vi "BStAT_(Doubles).vi"() -> ()   [LabVIEW 2013]
uses:
  <vilib>/Utility/file.llb/Read From Spreadsheet File (DBL).vi
  <vilib>/Utility/file.llb/Write To Spreadsheet File (I64).vi
panel:
  out "framesPerSecond":u32
  out "serve to point":dbl[](array[numeric])
  in  "Word._Application":refnum<k7>
  out "p2y":dbl[](array[numeric])
  out "p1y":dbl[](array[numeric])
  out "point frames":dbl[](array[numeric])
  out "service frames":dbl[](array[numeric])
  out "comp_p1 2":dbl[](array[numeric])
  out "comp_p2 2":dbl[](array[numeric])
  out "comp_p2":dbl[](array[numeric])
  out "comp_p1":dbl[](array[numeric])
  out "game":i32[][](array[numeric])
  out "save2_data":dbl[][](array[numeric])
  out "save1_data":dbl[][](array[numeric])
  out "save2":i32[][](array[numeric])
  out "save1":i32[][](array[numeric])
  out "filedata in":dbl[][](array[numeric]) format="%0.3f"
  out "edited\nevents":dbl[][](array[numeric])
  out "edited to play":dbl[](array[numeric])
  out "P2 position":bool
  out "P1 position":bool
  out "p2code":i32
  out "p1code":i32
  out "frames":dbl[](array[numeric])
  out "Events":bool[](array[boolean])
  out "coded data":dbl[][](array[numeric])
  out "frame data":dbl[][](array[numeric])
  out "Score":dbl[][](array[numeric])
  out "OH":bool[](array[boolean])
  out "BH":bool[](array[boolean])
  out "FH":bool[](array[boolean])
  in  "stop":bool
  in  "Tab Control":enum32{"Coding", "Display"}(tab)=enum."Display"
  in  "Name 4":string
  in  "Player 4":bool
  in  "Name 3":string
  in  "Player 3":bool
  in  "Name 2":string
  in  "Player 2":bool
  in  "Name 1":string
  in  "Player 1":bool
  in  "10 6":bool
  in  "10 5":bool
  in  "10 3":bool
  in  "10 4":bool
  in  "10 2":bool
  in  "10":bool
  in  "9 6":bool
  in  "9 5":bool
  in  "9 3":bool
  in  "9 4":bool
  in  "9 2":bool
  in  "9":bool
  in  "5 6":bool
  in  "5 5":bool
  in  "5 3":bool
  in  "5 4":bool
  in  "5 2":bool
  in  "5":bool
  in  "1 6":bool
  in  "1 5":bool
  in  "1 3":bool
  in  "1 4":bool
  in  "1 2":bool
  in  "1":bool
  in  "2 6":bool
  in  "2 5":bool
  in  "2 3":bool
  in  "2 4":bool
  in  "2 2":bool
  in  "2":bool
  in  "3 6":bool
  in  "3 5":bool
  in  "3 3":bool
  in  "3 4":bool
  in  "3 2":bool
  in  "3":bool
  in  "4 6":bool
  in  "4 5":bool
  in  "4 3":bool
  in  "4 4":bool
  in  "4 2":bool
  in  "4":bool
  in  "6 6":bool
  in  "6 5":bool
  in  "6 3":bool
  in  "6 4":bool
  in  "6 2":bool
  in  "6":bool
  in  "7 6":bool
  in  "7 5":bool
  in  "7 3":bool
  in  "7 4":bool
  in  "7 2":bool
  in  "7":bool
  in  "8 6":bool
  in  "8 5":bool
  in  "8 3":bool
  in  "8 4":bool
  in  "8 2":bool
  in  "8":bool
  in  "5":bool
  in  "TCL 3":bool
  in  "BCL 3":bool
  in  "MCL 3":bool
  in  "BCR 3":bool
  in  "MCR  3":bool
  in  "TCR 3":bool
  in  "TCL 2":bool
  in  "BCL 2":bool
  in  "MCL 2":bool
  in  "BCR 2":bool
  in  "MCR 2":bool
  in  "TCR 2":bool
  in  "Drag control":u32(slide) min=400 max=3000 scale=0.0..6446.0
  in  "UNDO":bool
  out "Last coded":i32
  in  "Progress...":i32(slide) min=400 max=3000 scale=0.0..6277.0
  in  "1":bool
  in  "E2":bool
  in  "E1":bool
  in  "Score2":i32
  in  "W2":bool
  in  "W1":bool
  in  "Score1":i32
  in  "Pause 2":bool
  in  "F_Fr":bool
  in  "S_Fr":bool
  out "Video":T1(plugin-control)
  in  "START":bool
  in  "Video file":path caption="Open AVI file"
  in  "Save data":path caption="Save data to file (select folder ONLY)"
  in  "Start Coding":bool
  out "F_frame":u32
  out "S_frame":u32
  in  "playback speed":dbl(slide) step=0.25 scale=0.25..4.0
  in  "fast forward":bool
  in  "TL 2":bool
  in  "BR 2":bool
  in  "BL 2":bool
  in  "BC 2":bool
  in  "MR  2":bool
  in  "MC 2":bool
  in  "ML 2":bool
  in  "TR 2":bool
  in  "TC 2":bool
  in  "TL 3":bool
  in  "BR 3":bool
  in  "BL 3":bool
  in  "BC 3":bool
  in  "MR  3":bool
  in  "MC 3":bool
  in  "ML 3":bool
  in  "TR 3":bool
  in  "TC 3":bool
  in  "Pause 1":bool
  out "coding":i32[][](array[numeric])
  in  "S2":bool
  in  "S1":bool
  in  "2":bool
  in  "3":bool
  in  "4":bool
  in  "Pause 3":bool
  in  "switch sides":bool
  in  "S3":bool
  in  "S4":bool
  in  "Stop and save":bool
  out "Numeric":dbl format="%<%H:%M:%S>t"
  in  "play back":i32(slide)=1 min=0 max=101 scale=0.0..101.0
  out "DISP":T1(plugin-control)
  in  "Vid file":path caption="Open AVI file"
  in  "Data file":path caption="Read data from"
  in  "Tab Control 2":enum32{"Edit ", "Data Display", "Momentum"}(tab)
  in  "5 2":bool
  in  "1 2":bool
  in  "Serve2":bool
  in  "Serve1":bool
  in  "2 2":bool
  in  "3 2":bool
  in  "4 2":bool
  in  "Serve3":bool
  in  "Serve4":bool
  in  "TCL 4":bool
  in  "BCL 4":bool
  in  "MCL 4":bool
  in  "BCR 4":bool
  in  "MCR  4":bool
  in  "TCR 4":bool
  in  "TL 4":bool
  in  "BR 4":bool
  in  "BL 4":bool
  in  "BC 4":bool
  in  "MR  4":bool
  in  "MC 4":bool
  in  "ML 4":bool
  in  "TR 4":bool
  in  "TC 4":bool
  in  "shots":u8(slide)=2 scale=0.0..5.0
  in  "point 2":bool
  in  "Rally":bool
  in  "Write VI":path caption="Write to AVI file"
  in  "before":u8(slide)=2
  in  "Playback Speed":dbl(slide)=1.0 min=0.25 max=30.0 step=0.25 scale=0.25..2.0
  in  "pause":bool
  in  "stop 2":bool
  in  "Playback\nscore":bool
  in  "P2 score":dbl
  in  "P1 score":dbl
  in  "error":bool
  in  "winner":bool
  in  "point 1":bool
  in  "Team1":bool
  in  "Team2":bool
  in  "FH 2":bool
  in  "BH 2":bool
  in  "ST":bool
  in  "CR 2":bool
  in  "clear":bool
  in  "lob":bool
  in  "drive":bool
  in  "smash":bool
  in  "DR defense":bool
  in  "Half Smash":bool
  in  "drop":bool
  in  "net":bool
  in  "OH 2":bool
  in  "Play":bool
  in  "after":u8(slide)=2 scale=0.0..5.0
  in  "write file":bool
  out "Search events":i32(slide) caption="Scaning(events)..." min=400 max=3000 scale=0.0..86.0
  out "Search score":i32(slide) caption="Searching(score)..." min=400 max=3000 scale=0.0..35.0
  out "writing":i32(slide) caption="Writing..." min=400 max=3000 scale=0.0..101.0
  in  "3 shots":bool
  in  "CL defense":bool
  in  "BL defense":bool
  in  "Player 32":bool
  in  "Player 12":bool
  in  "Player 22":bool
  in  "Player 42":bool
  in  "Compare":bool
  in  "2":string(combo)="1"
  in  "1":string(combo)="1"
  in  "save2":string
  in  "save1":string
  in  "save2":bool
  in  "save1":bool
  in  "Percentage":bool
  in  "display\nselection":string(combo)="1"
  in  "To make white":enum32{""}(tab)
  out "p2 23":string
  out "p2 22":string
  out "p2 21":string
  out "p2 20":string
  out "p2 19":string
  out "p2 18":string
  out "p1 15":string
  out "p1 14":string
  out "p1 13":string
  out "p1 12":string
  out "p1 11":string
  out "p1 10":string
  out "p2 17":string
  out "p2 16":string
  out "p2 11":string
  out "p2 10":string
  out "p2 9":string
  out "p2 14":string
  out "p2 13":string
  out "p2 12":string
  out "p2 15":string
  out "p1 5":string
  out "p1 7":string
  out "p1 6":string
  out "p1 4":string
  out "p1 1":string
  out "p1 3":string
  out "p1 2":string
  out "p1 8":string
  out "p1 9":string
  out "player1 2":string[](array[string])=["0", "0", "0", "0", "0", "0", "0", "0", "0", "0"]
  out "P1graph":cluster{dbl[], "array":dbl[]}(graph)={[0.0, nan, 0.0, nan, 0.0, nan, 0.0, nan, 0.0, nan, 0.0, nan, 0.0, nan, 0.0, nan, 0.0], "array"=[1.0, 2.0, 3.0, 4.0, 5.0, 6.0, 7.0, 8.0, 9.0, 10.0, 11.0, 12.0, 13.0, 14.0, 15.0, 16.0, 17.0]}
  out "Player 1":string[](array[string])=["Fore hand", "Back hand", "Over head", "", "Straight", "Cross", "", "Smash", "Half smash", "DRIVE DEF", "BLOCK DEF", "CLEAR DEF", "Drive/Tap", "Lob", "Drop", "Clear", "Net"]
  out "player2 2":string[](array[string])=["0", "0", "0", "0", "0", "0", "0", "0", "0", "0"]
  out "P2graph":cluster{dbl[], "array":dbl[]}(graph)={[0.0, nan, 0.0, nan, 0.0, nan, 0.0, nan, 0.0, nan, 0.0, nan, 0.0, nan, 0.0, nan, 0.0], "array"=[1.0, 2.0, 3.0, 4.0, 5.0, 6.0, 7.0, 8.0, 9.0, 10.0, 11.0, 12.0, 13.0, 14.0, 15.0, 16.0, 17.0]}
  out "Player 2":string[](array[string])=["Fore hand", "Back hand", "Over head", "", "Straight", "Cross", "", "Smash", "Half smash", "DRIVE DEF", "BLOCK DEF", "CLEAR DEF", "Drive/Tap", "Lob", "Drop", "Clear", "Net"]
  out "W1/E1":string[](array[string])=["0", "0"]
  out "W2/E2":string[](array[string])=["0", "0"]
  out "W/E2":string[](array[string])=["Fore hand", "Back hand", "Over head", "", "Strainght", "Cross", "", "Lob", "Clear", "Drive", "Smash", "Defence", "Chop", "Drop", "Net"]
  out "W/E1":string[](array[string])=["Fore hand", "Back hand", "Over head", "", "Strainght", "Cross", "", "Lob", "Clear", "Drive", "Smash", "Defence", "Chop", "Drop", "Net"]
  out "player2_2":string[](array[string])=["0", "0", "0", "", "0", "0"]
  out "player1_2":string[](array[string])=["0", "0", "0", "", "0", "0"]
  out "Player 2_2":string[](array[string])=["Fore hand", "Back hand", "Over head", "", "Strainght", "Cross", "", "Lob", "Clear", "Drive", "Smash", "Defence", "Chop", "Drop", "Net"]
  out "Player 1_2":string[](array[string])=["Fore hand", "Back hand", "Over head", "", "Strainght", "Cross", "", "Lob", "Clear", "Drive", "Smash", "Defence", "Chop", "Drop", "Net"]
  in  "to make white 2":enum32{""}(tab)
  out "Shortest rally length(sec)":dbl format="%#_3g"
  out "Longest rally length(sec)":dbl format="%#_3g"
  out "momentum graph":cluster{dbl[], dbl[]}[](graph)
  out "Score":dbl[](array[numeric])
  out "Average rally length(sec)":dbl format="%#_3g"
  out "Rally length(sec)":dbl format="%#_3g"
  in  "edit video":bool
  in  "REPORT":bool
  # "Strategic Analysis Tool for Badminton"
  # "Position"
  # "Score"
  # "Smash"
  # "Half Smash"
  # "DRIVE Defence"
  # "BLOCK Defence"
  # "CLEAR Defence"
  # "Drive/Tap"
  # "Lob"
  # "Drop"
  # "Clear"
  # "Net"
  # "Overhead"
  # "Straight"
  # "Cross"
  # "Forehand"
  # "Straight"
  # "Cross"
  # "Backhand"
  # "Straight"
  # "Cross"
  # "Shots to Playback"
  # "TEAM / Player"
  # "Position"
  # "Special Events"
  # "Playback interval (s)"
  # "Score"
  # "to"
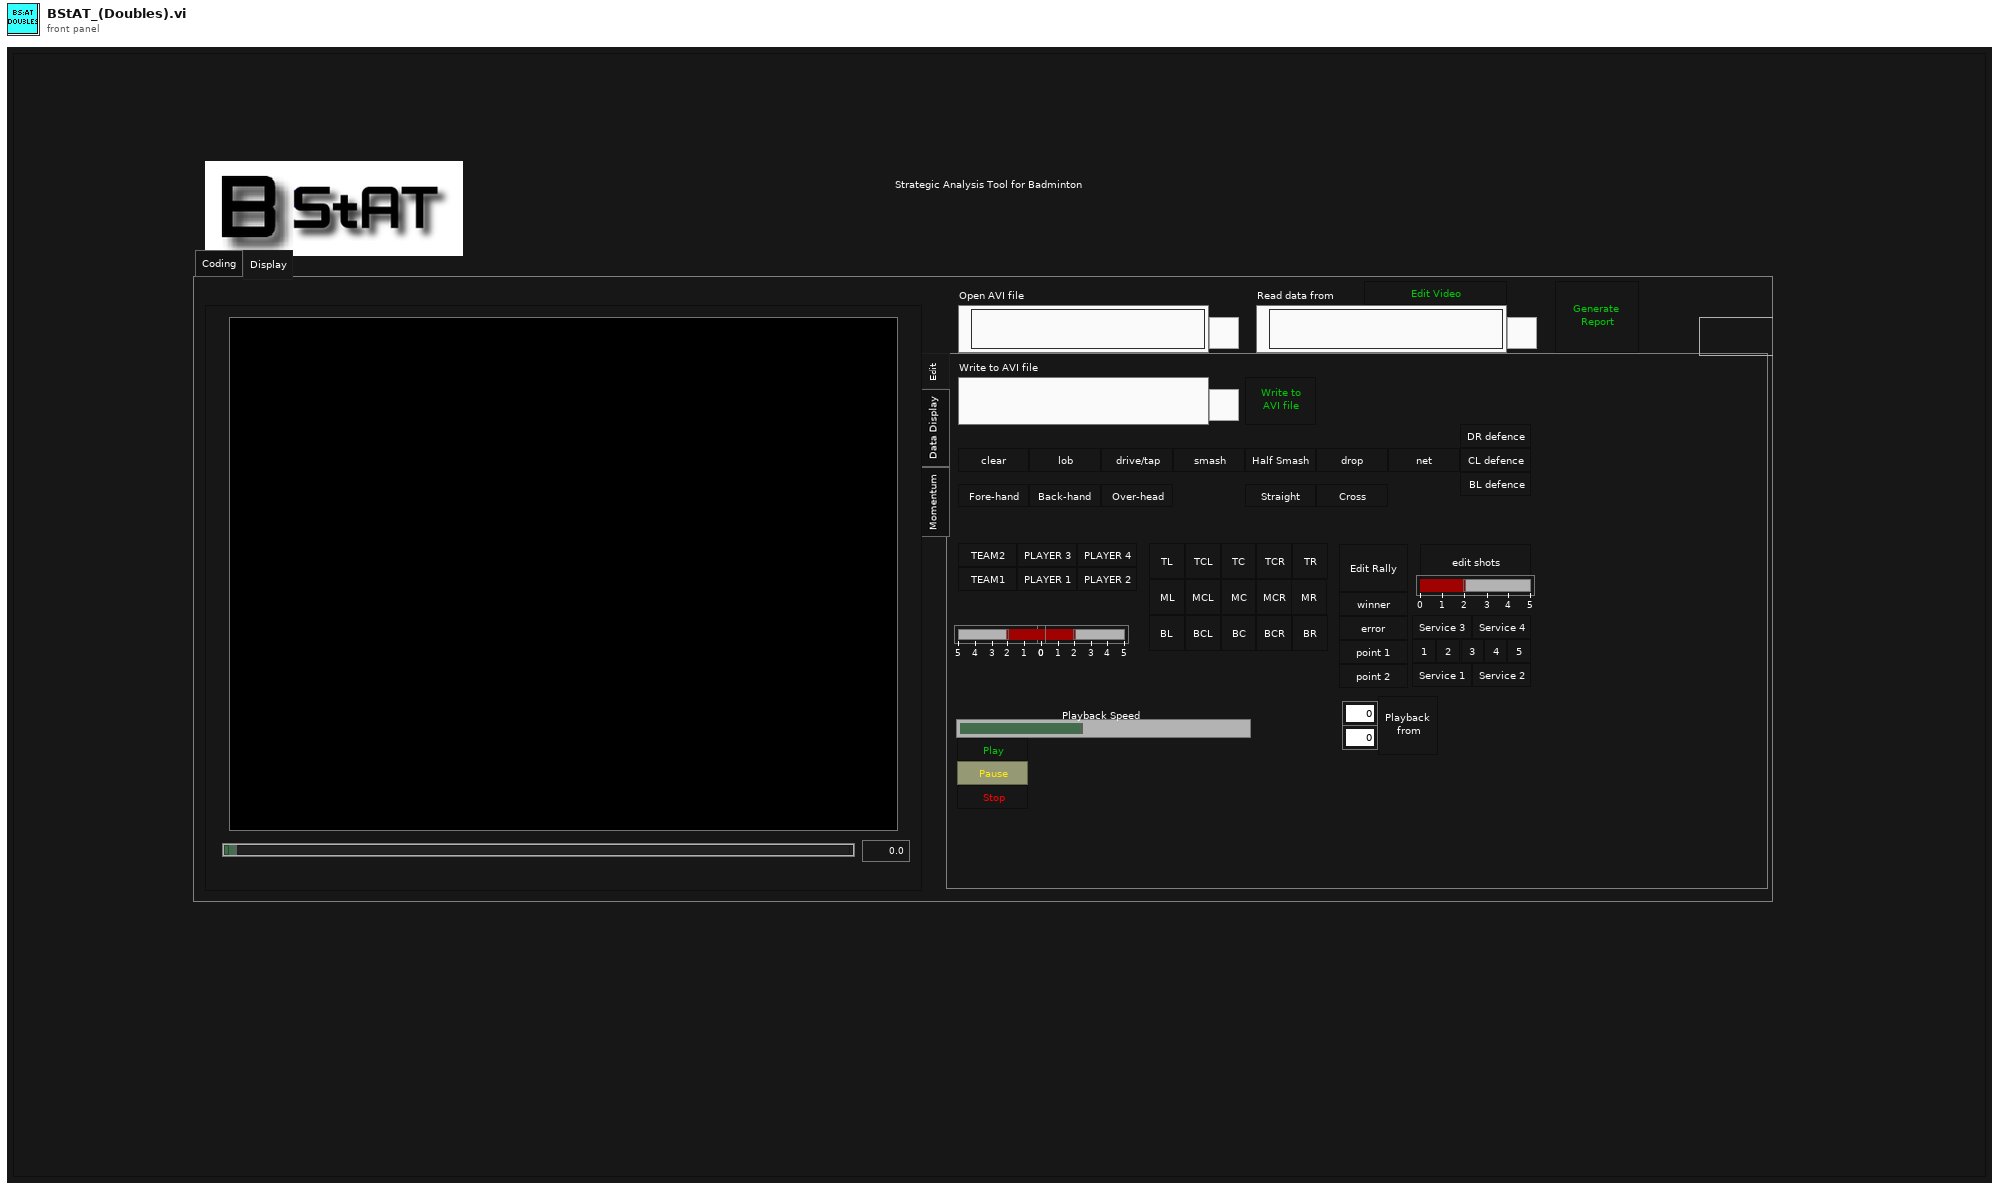
[diagram p1: front panel]
types:
  T1 = typedef "IMAQ Image.ctl" = refnum<image>
  T2 = enum8{"Enabled", "Disabled", "Disabled and Grayed Out"}
  T3 = enum16{"open", "replace", "create", "open or create", "replace or create", "replace or create with confirmation"}
  T4 = typedef "Image Type" = u32
  T5 = typedef "AviRefnum.ctl" = refnum<k1>
  T6 = cluster{"width":u32, "height":u32, "framesPerSecond":u32, "compressionFilter":string, "hasData":bool}
  T7 = typedef "LVPositionTypeDef.ctl" = cluster{"Left":i32, "Top":i32}
  T8 = cluster{"Position":T7, "Position":T7, "Position":T7, "Position":T7, "Position":T7, "Position":T7, "Position":T7, "Position":T7}
  T9 = cluster{"Position":T7, "Position":T7, "Position":T7, "Position":T7, "Position":T7, "Position":T7}
  T10 = cluster{"Position":T7, "Position":T7, "Position":T7, "Position":T7}
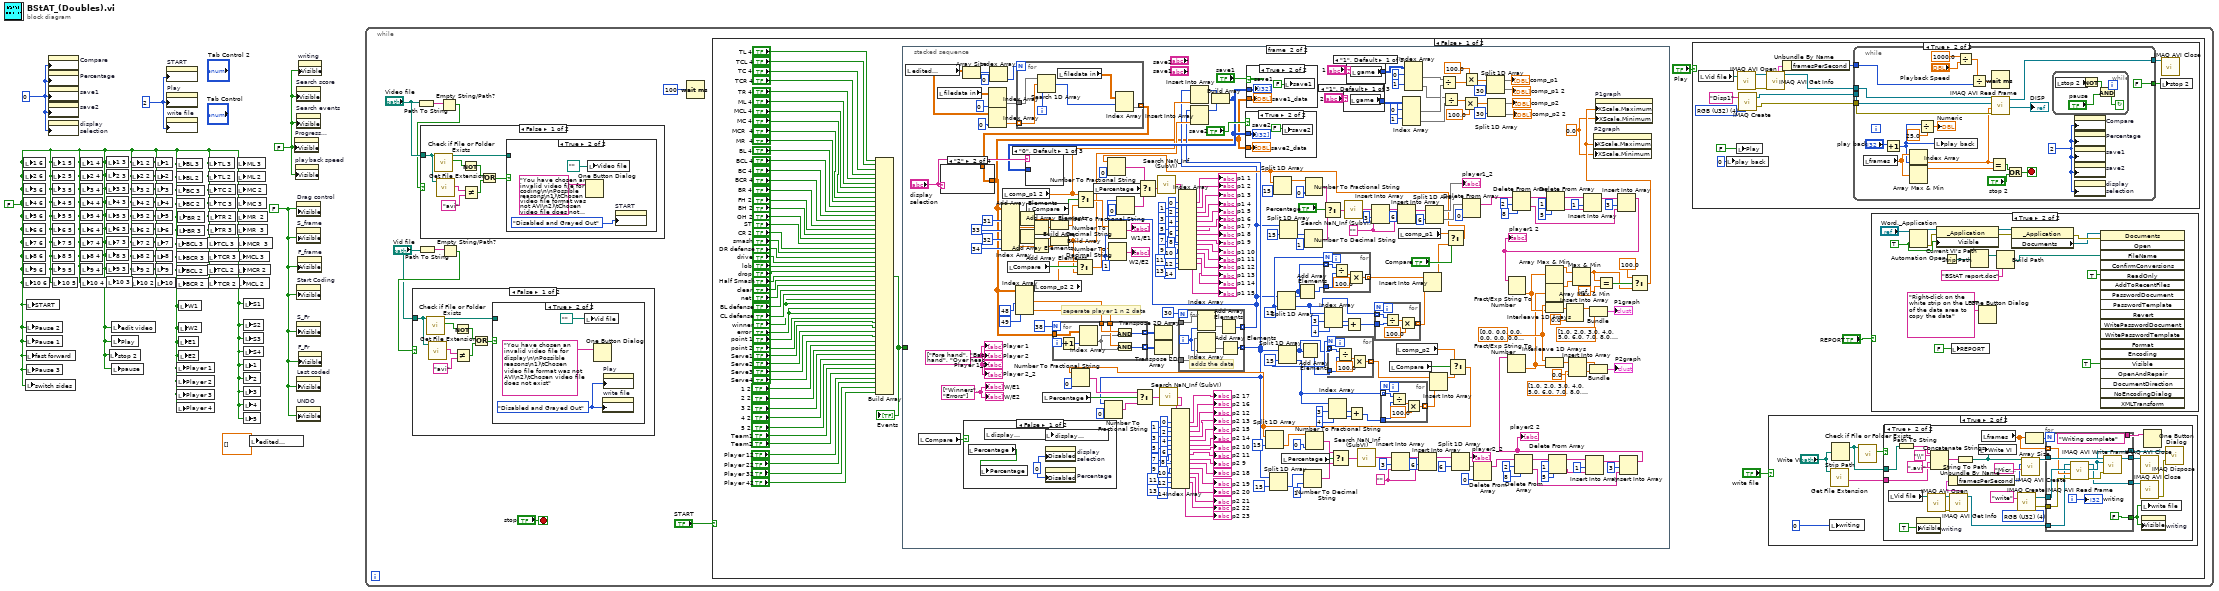
[diagram p0: block diagram]
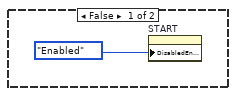
[diagram p2: hidden frame]
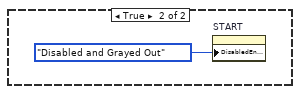
[diagram p3: hidden frame]
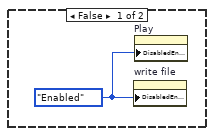
[diagram p4: hidden frame]
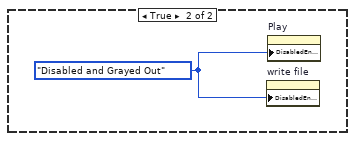
[diagram p5: hidden frame]
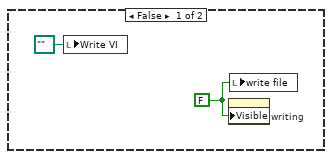
[diagram p7: hidden frame]
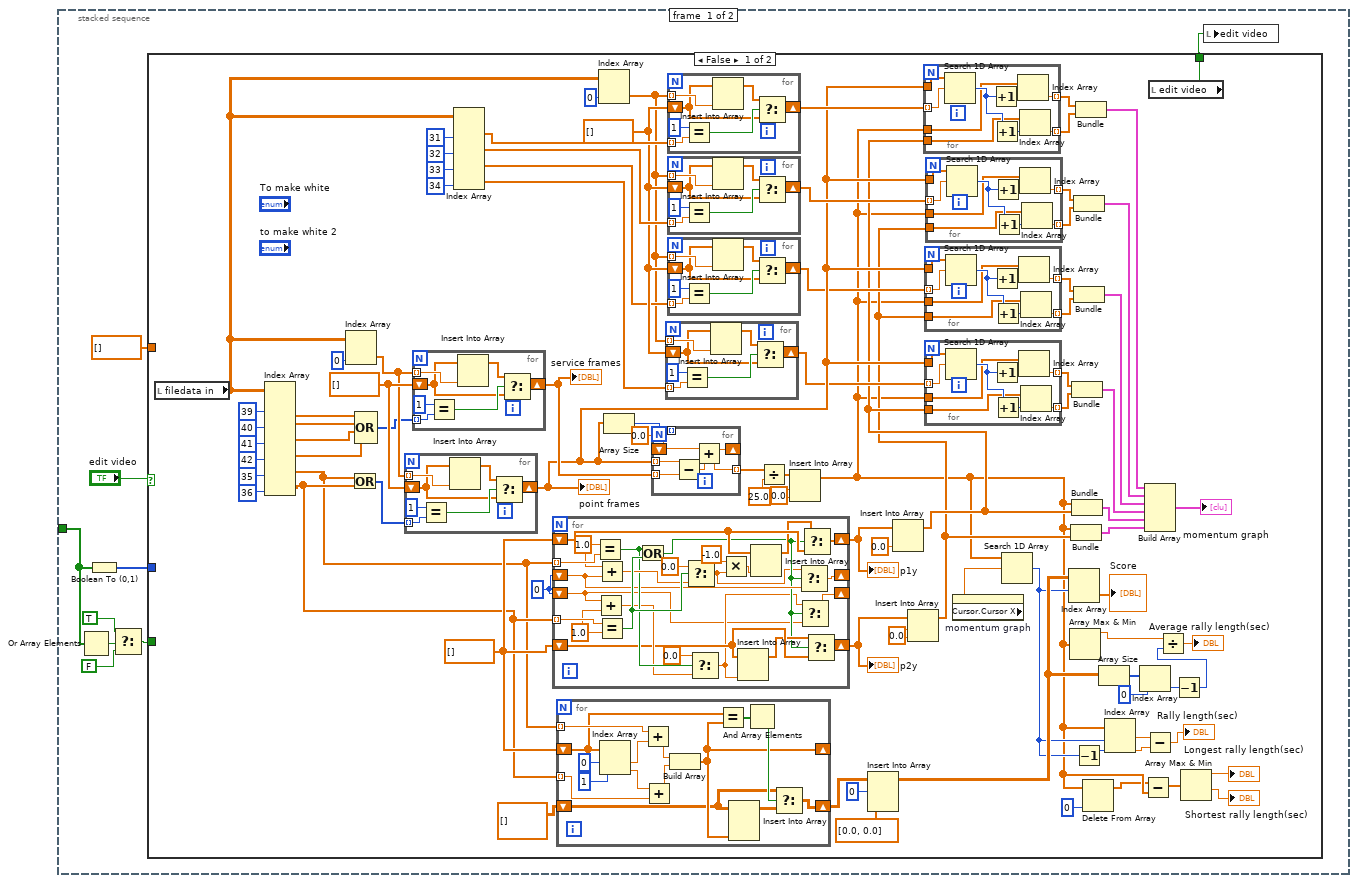
[diagram p9: hidden frame]
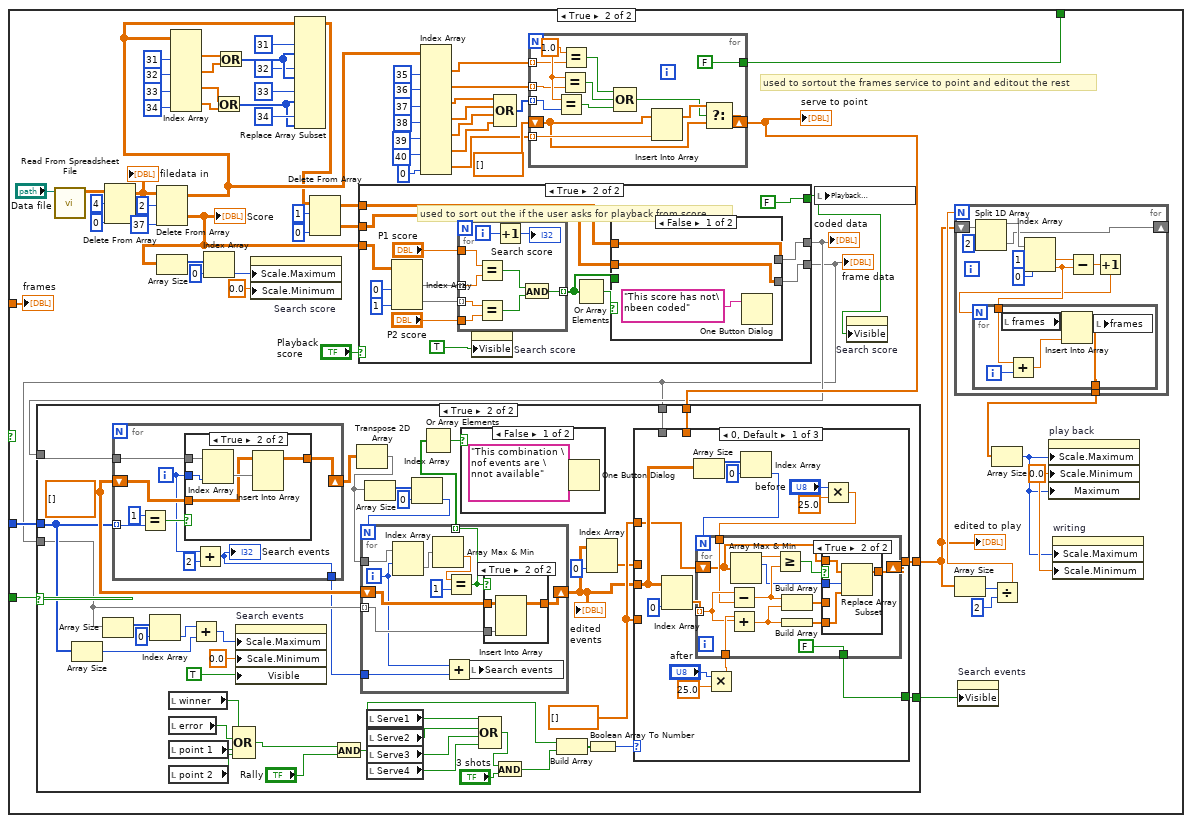
[diagram p10: hidden frame]
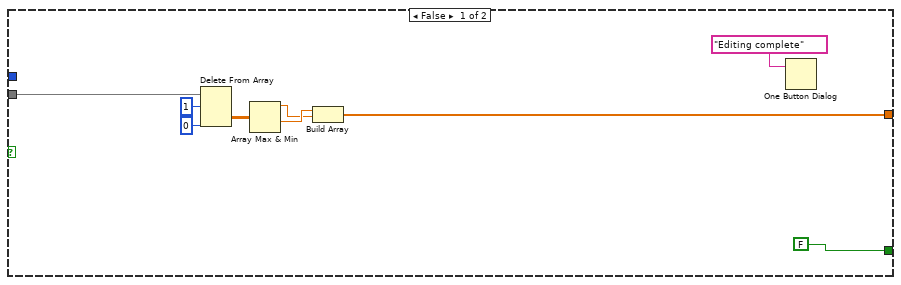
[diagram p11: hidden frame]
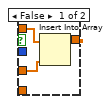
[diagram p12: hidden frame]
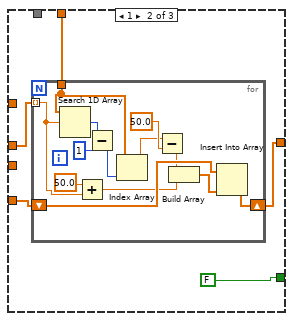
[diagram p13: hidden frame]
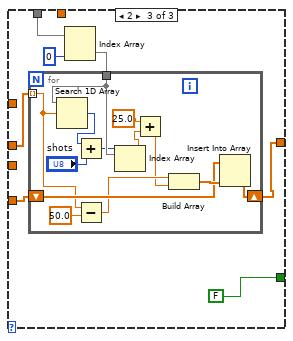
[diagram p14: hidden frame]
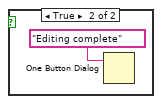
[diagram p15: hidden frame]
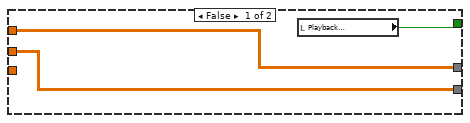
[diagram p18: hidden frame]
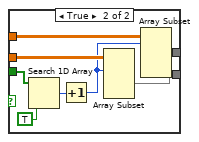
[diagram p19: hidden frame]
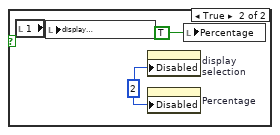
[diagram p20: hidden frame]
diagram:
  w1 = 2 ("play back")
  w2 = 0 ("play back")
  w3 = FALSE ("4 6")
  w4 = FALSE ("Visible")
  w5 = FALSE ("Visible")
  n1 = local write "1 6"(w3) -> ()
  n2 = local write "2 6"(w3) -> ()
  n3 = local write "3 6"(w3) -> ()
  n4 = local write "4 6"(w3) -> ()
  n5 = local write "5 6"(w3) -> ()
  n6 = local write "6 6"(w3) -> ()
  n7 = local write "7 6"(w3) -> ()
  n8 = local write "8 6"(w3) -> ()
  n9 = local write "9 6"(w3) -> ()
  n10 = local write "10 6"(w3) -> ()
  n11 = local write "switch sides"(w3) -> ()
  n12 = local write "START"(w3) -> ()
  n13 = local write "Pause 2"(w3) -> ()
  n14 = local write "Pause 1"(w3) -> ()
  n15 = local write "fast forward"(w3) -> ()
  n16 = local write "Pause 3"(w3) -> ()
  n17 = property on="Compare" class="Bool (strict)"("DisabledEnum"=w2) -> ()  [unwired: 2 in, 2 out]
  n18 = property on="Percentage" class="Bool (strict)"("DisabledEnum"=w2) -> ()  [unwired: 2 in, 2 out]
  n19 = property on="save1" class="Bool (strict)"("DisabledEnum"=w2) -> ()  [unwired: 2 in, 2 out]
  n20 = property on="save2" class="Bool (strict)"("DisabledEnum"=w2) -> ()  [unwired: 2 in, 2 out]
  n21 = property on="display\nselection" class="CmbBox"("DisabledEnum"=w2) -> ()  [unwired: 2 in, 2 out]
  n22 = local write "1 5"(w3) -> ()
  n23 = local write "2 5"(w3) -> ()
  n24 = local write "3 5"(w3) -> ()
  n25 = local write "4 5"(w3) -> ()
  n26 = local write "5 5"(w3) -> ()
  n27 = local write "6 5"(w3) -> ()
  n28 = local write "7 5"(w3) -> ()
  n29 = local write "8 5"(w3) -> ()
  n30 = local write "9 5"(w3) -> ()
  n31 = local write "10 5"(w3) -> ()
  n32 = local write "1 4"(w3) -> ()
  n33 = local write "2 4"(w3) -> ()
  n34 = local write "3 4"(w3) -> ()
  n35 = local write "4 4"(w3) -> ()
  n36 = local write "5 4"(w3) -> ()
  n37 = local write "6 4"(w3) -> ()
  n38 = local write "7 4"(w3) -> ()
  n39 = local write "8 4"(w3) -> ()
  n40 = local write "9 4"(w3) -> ()
  n41 = local write "10 4"(w3) -> ()
  n42 = local write "1 3"(w3) -> ()
  n43 = local write "2 3"(w3) -> ()
  n44 = local write "3 3"(w3) -> ()
  n45 = local write "4 3"(w3) -> ()
  n46 = local write "5 3"(w3) -> ()
  n47 = local write "6 3"(w3) -> ()
  n48 = local write "7 3"(w3) -> ()
  n49 = local write "8 3"(w3) -> ()
  n50 = local write "9 3"(w3) -> ()
  n51 = local write "10 3"(w3) -> ()
  n52 = local write "stop 2"(w3) -> ()
  n53 = local write "edit video"(w3) -> ()
  n54 = local write "Play"(w3) -> ()
  n55 = local write "pause"(w3) -> ()
  n56 = local write "1 2"(w3) -> ()
  n57 = local write "2 2"(w3) -> ()
  n58 = local write "3 2"(w3) -> ()
  n59 = local write "4 2"(w3) -> ()
  n60 = local write "5 2"(w3) -> ()
  n61 = local write "6 2"(w3) -> ()
  n62 = local write "7 2"(w3) -> ()
  n63 = local write "8 2"(w3) -> ()
  n64 = local write "9 2"(w3) -> ()
  n65 = local write "10 2"(w3) -> ()
  n66 = local write "1"(w3) -> ()
  n67 = local write "2"(w3) -> ()
  n68 = local write "3"(w3) -> ()
  n69 = local write "4"(w3) -> ()
  n70 = local write "5"(w3) -> ()
  n71 = local write "6"(w3) -> ()
  n72 = local write "7"(w3) -> ()
  n73 = local write "8"(w3) -> ()
  n74 = local write "9"(w3) -> ()
  n75 = local write "10"(w3) -> ()
  n76 = property on="START" class="Bool (strict)"("DisabledEnum"=w1) -> ()  [unwired: 2 in, 2 out]
  n77 = property on="Play" class="Bool (strict)"("DisabledEnum"=w1) -> ()  [unwired: 2 in, 2 out]
  n78 = property on="write file" class="Bool (strict)"("DisabledEnum"=w1) -> ()  [unwired: 2 in, 2 out]
  n79 = local write "BCL 3"(w3) -> ()
  n80 = local write "BCL 2"(w3) -> ()
  n81 = local write "BL 3"(w3) -> ()
  n82 = local write "BL 2"(w3) -> ()
  n83 = local write "BC 3"(w3) -> ()
  n84 = local write "BC 2"(w3) -> ()
  n85 = local write "BCR 3"(w3) -> ()
  n86 = local write "BCR 2"(w3) -> ()
  n87 = local write "Player 1"(w3) -> ()
  n88 = local write "Player 2"(w3) -> ()
  n89 = local write "Player 3"(w3) -> ()
  n90 = local write "Player 4"(w3) -> ()
  n91 = local write "BR 2"(w3) -> ()
  n92 = local write "BR 3"(w3) -> ()
  n93 = local write "W1"(w3) -> ()
  n94 = local write "W2"(w3) -> ()
  n95 = local write "E1"(w3) -> ()
  n96 = local write "E2"(w3) -> ()
  n97 = local write "TCL 3"(w3) -> ()
  n98 = local write "TCL 2"(w3) -> ()
  n99 = local write "TL 3"(w3) -> ()
  n100 = local write "TL 2"(w3) -> ()
  n101 = local write "TC 2"(w3) -> ()
  n102 = local write "TC 3"(w3) -> ()
  n103 = local write "TCR 3"(w3) -> ()
  n104 = local write "TCR 2"(w3) -> ()
  n105 = local write "TR 2"(w3) -> ()
  n106 = local write "TR 3"(w3) -> ()
  n107 = local write "MCL 3"(w3) -> ()
  n108 = local write "MCL 2"(w3) -> ()
  n109 = local write "ML 3"(w3) -> ()
  n110 = local write "ML 2"(w3) -> ()
  n111 = local write "MC 2"(w3) -> ()
  n112 = local write "MC 3"(w3) -> ()
  n113 = local write "MR  2"(w3) -> ()
  n114 = local write "MR  3"(w3) -> ()
  n115 = local write "MCR  3"(w3) -> ()
  n116 = local write "MCR 2"(w3) -> ()
  n117 = local write "S1"(w3) -> ()
  n118 = local write "S2"(w3) -> ()
  n119 = local write "S3"(w3) -> ()
  n120 = local write "S4"(w3) -> ()
  n121 = local write "1"(w3) -> ()
  n122 = local write "2"(w3) -> ()
  n123 = local write "3"(w3) -> ()
  n124 = local write "4"(w3) -> ()
  n125 = local write "5"(w3) -> ()
  n126 = local write "edited\nevents"(dbl[][] []) -> ()
  n127 = property on="Progress..." class="Slide (strict)"("Visible"=w5) -> ()  [unwired: 2 in, 2 out]
  n128 = property on="playback speed" class="Slide (strict)"("Visible"=w5) -> ()  [unwired: 2 in, 2 out]
  n129 = property on="Search score" class="Slide (strict)"("Visible"=w5) -> ()  [unwired: 2 in, 2 out]
  n130 = property on="Search events" class="Slide (strict)"("Visible"=w5) -> ()  [unwired: 2 in, 2 out]
  n131 = property on="Drag control" class="Slide (strict)"("Visible"=w4) -> ()  [unwired: 2 in, 2 out]
  n132 = property on="S_frame" class="DigNum (strict)"("Visible"=w4) -> ()  [unwired: 2 in, 2 out]
  n133 = property on="Start Coding" class="Bool (strict)"("Visible"=w4) -> ()  [unwired: 2 in, 2 out]
  n134 = property on="S_Fr" class="Bool (strict)"("Visible"=w4) -> ()  [unwired: 2 in, 2 out]
  n135 = property on="Last coded" class="DigNum (strict)"("Visible"=w4) -> ()  [unwired: 2 in, 2 out]
  n136 = property on="UNDO" class="Bool (strict)"("Visible"=w4) -> ()  [unwired: 2 in, 2 out]
  n137 = property on="F_frame" class="DigNum (strict)"("Visible"=w4) -> ()  [unwired: 2 in, 2 out]
  n138 = property on="writing" class="Slide (strict)"("Visible"=w5) -> ()  [unwired: 2 in, 2 out]
  n139 = property on="F_Fr" class="Bool (strict)"("Visible"=w4) -> ()  [unwired: 2 in, 2 out]
  n140 = while {
    stop <- "stop" stop-if-true
    n141 = Path To String(path="Video file") -> (string=w9:string)
    n142 = Path To String(path="Vid file") -> (string=w12:string)
    n143 = Empty String/Path?(string/path=w9) -> (empty?=w7:bool)
    n144 = case shown="False" w7 {
      tunnel: "Video file" -> [w23 _]
      frame False {
        n145 = call <vilib>:"Check if File or Folder Exists.vi"("path"=w23) -> ("file or folder exists?"=w18:bool, "dup path"=w19:path)  [unwired: 8 in, 1 out]
        n146 = call <vilib>:"Get File Extension.vi"("file"=w23) -> ("lowercase file extension"=w22:string)  [unwired: 7 in, 3 out]
        n147 = Not(x=w18) -> (.not. x?=w17:bool)
        n148 = Not Equal?(x=w22, y="avi" ("lowercase file extension")) -> (x != y?=w21:bool)
        n149 = Or(x=w17, y=w21) -> (x .or. y?=w20:bool)
        n150 = case shown="True" w20 {
          tunnel: w19 -> [_ _]
          frame False {
            n151 = property on="START" class="Bool (strict)"("DisabledEnum"=T2."Enabled" ("Disabled")) -> ()  [unwired: 2 in, 2 out]
          }
          frame True {
            n152 = One Button Dialog(message="You have chosen an invalid video file for coding\n\nPossible reasons\n1)\tChosen video file format was not AVI\n2)\tChosen video file does not exist") -> ()  [unwired: 1 in, 1 out]
            n153 = local write "Video file"(path "" ("Video file")) -> ()
            n154 = property on="START" class="Bool (strict)"("DisabledEnum"=T2."Disabled and Grayed Out" ("Disabled")) -> ()  [unwired: 2 in, 2 out]
          }
        }
      }
      frame True {
        n155 = property on="START" class="Bool (strict)"("DisabledEnum"=T2."Disabled and Grayed Out" ("Disabled")) -> ()  [unwired: 2 in, 2 out]
      }
    }
    n156 = Empty String/Path?(string/path=w12) -> (empty?=w11:bool)
    n157 = case shown="False" w11 {
      tunnel: "Vid file" -> [w36 _]
      frame False {
        n158 = call <vilib>:"Check if File or Folder Exists.vi"("path"=w36) -> ("file or folder exists?"=w30:bool, "dup path"=w31:path)  [unwired: 8 in, 1 out]
        n159 = call <vilib>:"Get File Extension.vi"("file"=w36) -> ("lowercase file extension"=w35:string)  [unwired: 7 in, 3 out]
        n160 = Not(x=w30) -> (.not. x?=w29:bool)
        n161 = Not Equal?(x=w35, y="avi" ("lowercase file extension")) -> (x != y?=w33:bool)
        n162 = Or(x=w29, y=w33) -> (x .or. y?=w32:bool)
        n163 = case shown="True" w32 {
          tunnel: w31 -> [_ _]
          frame False {
            w37 = T2."Enabled" ("Disabled")
            n164 = property on="write file" class="Bool (strict)"("DisabledEnum"=w37) -> ()  [unwired: 2 in, 2 out]
            n165 = property on="Play" class="Bool (strict)"("DisabledEnum"=w37) -> ()  [unwired: 2 in, 2 out]
          }
          frame True {
            w39 = T2."Disabled and Grayed Out" ("Disabled")
            n166 = local write "Vid file"(path "" ("Video file")) -> ()
            n167 = One Button Dialog(message="You have chosen an invalid video file for display\n\nPossible reasons\n1)\tChosen video file format was not AVI\n2)\tChosen video file does not exist") -> ()  [unwired: 1 in, 1 out]
            n168 = property on="write file" class="Bool (strict)"("DisabledEnum"=w39) -> ()  [unwired: 2 in, 2 out]
            n169 = property on="Play" class="Bool (strict)"("DisabledEnum"=w39) -> ()  [unwired: 2 in, 2 out]
          }
        }
      }
      frame True {
        w41 = T2."Disabled and Grayed Out" ("Disabled")
        n170 = property on="write file" class="Bool (strict)"("DisabledEnum"=w41) -> ()  [unwired: 2 in, 2 out]
        n171 = property on="Play" class="Bool (strict)"("DisabledEnum"=w41) -> ()  [unwired: 2 in, 2 out]
      }
    }
    n172 = Wait (ms)(milliseconds to wait=u32 100) -> ()  [unwired: 1 out]
    n173 = case shown="False" "START" {
      frame False {
        n174 = Build Array("TL 4", "TCL 4", "TC 4", "TCR 4", "TR 4", "ML 4", "MCL 4", "MC 4", "MCR  4", "MR  4", "BL 4", "BCL 4", "BC 4", "BCR 4", "BR 4", "FH 2", "BH 2", "OH 2", "ST", "CR 2", "smash", "DR defense", "drive", "lob", "drop", "Half Smash", "clear", "net", "BL defense", "CL defense", "winner", "winner", "error", "error", "point 1", "point 2", "Serve1", "Serve2", "Serve3", "Serve4", "1 2", "2 2", "3 2", "4 2", "5 2", "Team1", "Team2", "Player 12", "Player 22", "Player 32", "Player 42") -> (w86:bool[])
        "Events" <- w86
        n175 = stacked-sequence {
          tunnel: w86 -> [w163 _]
          frame #0 {
            n176 = Or Array Elements(Boolean array=w163) -> (logical OR=w166:bool)
            n177 = Boolean To (0,1)(Boolean=w163) -> (0, 1=w162:i16[])
            n178 = Select(t=TRUE, s=w166, f=FALSE) -> (s? t:f=w161:bool)
            n179 = case shown="False" "edit video" {
              tunnel: [w255 w391] -> w159
              tunnel: w162 -> [_ w389]
              tunnel: w161 -> [_ w427]
              tunnel: dbl[] [] ("edited\nto play 3") -> [_ w425]
              frame False {
                w211 = dbl[] []
                w245 = 0.0 ("new element/subarray")
                w244 = 0.0 ("new element/subarray")
                w243 = 0.0 ("new element/subarray")
                w195 = dbl[] []
                w196 = 0 ("disabled index (col)")
                w236 = dbl[] []
                n180 = local read "filedata in"() -> (w212:dbl[][])
                n181 = Index Array(array=w212, index (col) #1=39 ("length"), index (col) #2=40 ("disabled index (col)"), index (col) #3=41 ("index (col)"), index (col) #4=42 ("index (col)"), index (col) #5=35 ("index (col)"), index (col) #6=36 ("index (col)")) -> (element #1=w228:dbl[], element #2=w229:dbl[], element #3=w170:dbl[], element #4=w169:dbl[], element #5=w171:dbl[], element #6=w172:dbl[])  [unwired: 6 in]
                n182 = Index Array(array=w212, index (col)=0 ("disabled index (col)")) -> (element=w235:dbl[])  [unwired: 1 in]
                n183 = Or(x=w171, y=w172) -> (x .or. y?=w234:i32[])
                n184 = Compound Arithmetic op=OR(w228, w229, w170, w169) -> (w231:i32[])
                n185 = for {
                  tunnel: w234 -> [w372] mode=indexing
                  tunnel: w235 -> [w368] mode=indexing
                  shift-right: [w367] -> w207
                  shift-left: w236 -> [w366]
                  n186 = Equal?(x=1, y=w372) -> (x = y?=w370:bool)
                  n187 = Insert Into Array(array=w366, new element=w368) -> (w369:dbl[])  [unwired: 1 in]
                  n188 = Select(t=w369, s=w370, f=w366) -> (s? t:f=w367:dbl[])
                }
                "point frames" <- w207
                n189 = for {
                  tunnel: w231 -> [w379] mode=indexing
                  tunnel: w235 -> [w375] mode=indexing
                  shift-right: [w374] -> w238
                  shift-left: w236 -> [w373]
                  n190 = Equal?(x=1, y=w379) -> (x = y?=w377:bool)
                  n191 = Insert Into Array(array=w373, new element=w375) -> (w376:dbl[])  [unwired: 1 in]
                  n192 = Select(t=w376, s=w377, f=w373) -> (s? t:f=w374:dbl[])
                }
                "service frames" <- w238
                n193 = Index Array(array=w212, index (col) #1=31 ("disabled index (col)"), index (col) #2=32 ("index (col)"), index (col) #3=33 ("index (col)"), index (col) #4=34 ("index (col)")) -> (element #1=w221:dbl[], element #2=w222:dbl[], element #3=w210:dbl[], element #4=w209:dbl[])  [unwired: 4 in]
                n194 = for {
                  shift-right: [w264] -> _
                  shift-left: w196 -> [w263]
                  shift-right: [w260] -> _
                  shift-left: w196 -> [w259]
                  shift-right: [w269] -> w193
                  shift-left: w195 -> [w268]
                  shift-right: [w275] -> w194
                  shift-left: w195 -> [w266]
                  tunnel: w172 -> [w272] mode=indexing
                  tunnel: w171 -> [w280] mode=indexing
                  w271 = 1.0 ("x")
                  w277 = 1.0 ("x")
                  n195 = Equal?(x=w277, y=w280) -> (x = y?=w273:bool)
                  n196 = Add(x=w259, y=w271) -> (x+y=w270:dbl)
                  n197 = Add(x=w277, y=w263) -> (x+y=w276:dbl)
                  n198 = Equal?(x=w272, y=w271) -> (x = y?=w279:bool)
                  n199 = Or(x=w273, y=w279) -> (x .or. y?=w262:bool)
                  n200 = Select(t=0.0, s=w279, f=w276) -> (s? t:f=w256:dbl)
                  n201 = Select(t=0.0, s=w273, f=w270) -> (s? t:f=w261:dbl)
                  n202 = Multiply(x=-1.0 ("y"), y=w256) -> (x*y=w258:dbl)
                  n203 = Insert Into Array(array=w266, new element=w261) -> (w265:dbl[])  [unwired: 1 in]
                  n204 = Insert Into Array(array=w268, new element=w258) -> (w267:dbl[])  [unwired: 1 in]
                  n205 = Select(t=w256, s=w262, f=w263) -> (s? t:f=w264:dbl)
                  n206 = Select(t=w261, s=w262, f=w259) -> (s? t:f=w260:dbl)
                  n207 = Select(t=w267, s=w262, f=w268) -> (s? t:f=w269:dbl[])
                  n208 = Select(t=w265, s=w262, f=w266) -> (s? t:f=w275:dbl[])
                }
                "p1y" <- w193
                "p2y" <- w194
                n209 = for {
                  tunnel: w171 -> [w356] mode=indexing
                  tunnel: w172 -> [w352] mode=indexing
                  shift-right: [w348] -> _
                  shift-left: w195 -> [w351]
                  shift-right: [w346] -> w250
                  shift-left: dbl[][] [] -> [w345]
                  n210 = Index Array(array=w351, index #1=0 ("index"), index #2=1 ("index")) -> (element #1=w357:dbl, element #2=w355:dbl)
                  n211 = Add(x=w356, y=w357) -> (x+y=w354:dbl)
                  n212 = Add(x=w355, y=w352) -> (x+y=w353:dbl)
                  n213 = Build Array(w354, w353) -> (w348:dbl[])
                  n214 = Equal?(x=w351, y=w348) -> (x = y?=w350:bool[])
                  n215 = Insert Into Array(array=w345, new element=w348) -> (w347:dbl[][])  [unwired: 2 in]
                  n216 = And Array Elements(Boolean array=w350) -> (logical AND=w349:bool)
                  n217 = Select(t=w345, s=w349, f=w347) -> (s? t:f=w346:dbl[][])
                }
                n218 = Index Array(array=w212, index (col)=0 ("disabled index (col)")) -> (element=w208:dbl[])  [unwired: 1 in]
                n219 = Array Size(array=w207) -> (size(s)=w237:i32)
                n220 = for {
                  N: w237 -> [w360]
                  tunnel: w207 -> [w365] mode=indexing
                  tunnel: w238 -> [w364] mode=indexing
                  tunnel: [w361] -> w247 mode=indexing
                  shift-right: [w361] -> _
                  shift-left: 0.0 -> [w362]
                  tunnel: [w360] -> _ mode=indexing
                  n221 = Subtract(x=w365, y=w364) -> (x-y=w363:dbl)
                  n222 = Add(x=w362, y=w363) -> (x+y=w361:dbl)
                }
                n223 = for {
                  tunnel: w209 -> [w305] mode=indexing
                  tunnel: w208 -> [w301] mode=indexing
                  shift-right: [w300] -> w205
                  shift-left: w211 -> [w299]
                  n224 = Equal?(x=1, y=w305) -> (x = y?=w303:bool)
                  n225 = Insert Into Array(array=w299, new element=w301) -> (w302:dbl[])  [unwired: 1 in]
                  n226 = Select(t=w302, s=w303, f=w299) -> (s? t:f=w300:dbl[])
                }
                n227 = for {
                  tunnel: w221 -> [w344] mode=indexing
                  tunnel: w208 -> [w340] mode=indexing
                  shift-right: [w339] -> w218
                  shift-left: w211 -> [w338]
                  n228 = Equal?(x=1, y=w344) -> (x = y?=w342:bool)
                  n229 = Insert Into Array(array=w338, new element=w340) -> (w341:dbl[])  [unwired: 1 in]
                  n230 = Select(t=w341, s=w342, f=w338) -> (s? t:f=w339:dbl[])
                }
                n231 = for {
                  tunnel: w222 -> [w337] mode=indexing
                  tunnel: w208 -> [w333] mode=indexing
                  shift-right: [w332] -> w223
                  shift-left: w211 -> [w331]
                  n232 = Equal?(x=1, y=w337) -> (x = y?=w335:bool)
                  n233 = Insert Into Array(array=w331, new element=w333) -> (w334:dbl[])  [unwired: 1 in]
                  n234 = Select(t=w334, s=w335, f=w331) -> (s? t:f=w332:dbl[])
                }
                n235 = for {
                  tunnel: w210 -> [w312] mode=indexing
                  tunnel: w208 -> [w308] mode=indexing
                  shift-right: [w307] -> w206
                  shift-left: w211 -> [w306]
                  n236 = Equal?(x=1, y=w312) -> (x = y?=w310:bool)
                  n237 = Insert Into Array(array=w306, new element=w308) -> (w309:dbl[])  [unwired: 1 in]
                  n238 = Select(t=w309, s=w310, f=w306) -> (s? t:f=w307:dbl[])
                }
                n239 = Divide(x=w247, y=25.0 ("new element/subarray")) -> (x/y=w246:dbl[])
                n240 = Insert Into Array(array=w246, index=w243, new element=w243) -> (w177:dbl[])
                n241 = Insert Into Array(array=w250, index (row)=0, new element=dbl[] [0.0, 0.0] ("new element/subarray")) -> (w190:dbl[][])  [unwired: 1 in]
                n242 = Insert Into Array(array=w193, index=w245, new element=w245) -> (w192:dbl[])
                n243 = Insert Into Array(array=w194, index=w244, new element=w244) -> (w191:dbl[])
                n244 = for {
                  tunnel: w218 -> [w330] mode=indexing
                  tunnel: w207 -> [w329]
                  tunnel: [w327] -> w219 mode=indexing
                  tunnel: [w324] -> w220 mode=indexing
                  tunnel: w177 -> [w323]
                  tunnel: w192 -> [w322]
                  n245 = Search 1D Array(1D array=w329, element=w330) -> (index of element=w325:i32)  [unwired: 1 in]
                  n246 = Increment(x=w325) -> (x+1=w328:i32)
                  n247 = Increment(x=w325) -> (x+1=w326:i32)
                  n248 = Index Array(array=w323, index=w328) -> (element=w327:dbl)
                  n249 = Index Array(array=w322, index=w326) -> (element=w324:dbl)
                }
                n250 = for {
                  tunnel: w206 -> [w298] mode=indexing
                  tunnel: w207 -> [w297]
                  tunnel: [w295] -> w204 mode=indexing
                  tunnel: [w292] -> w203 mode=indexing
                  tunnel: w177 -> [w291]
                  tunnel: w191 -> [w290]
                  n251 = Search 1D Array(1D array=w297, element=w298) -> (index of element=w293:i32)  [unwired: 1 in]
                  n252 = Increment(x=w293) -> (x+1=w296:i32)
                  n253 = Increment(x=w293) -> (x+1=w294:i32)
                  n254 = Index Array(array=w291, index=w296) -> (element=w295:dbl)
                  n255 = Index Array(array=w290, index=w294) -> (element=w292:dbl)
                }
                n256 = for {
                  tunnel: w205 -> [w289] mode=indexing
                  tunnel: w207 -> [w288]
                  tunnel: [w286] -> w202 mode=indexing
                  tunnel: [w283] -> w201 mode=indexing
                  tunnel: w177 -> [w282]
                  tunnel: w192 -> [w281]
                  n257 = Search 1D Array(1D array=w288, element=w289) -> (index of element=w284:i32)  [unwired: 1 in]
                  n258 = Increment(x=w284) -> (x+1=w287:i32)
                  n259 = Increment(x=w284) -> (x+1=w285:i32)
                  n260 = Index Array(array=w282, index=w287) -> (element=w286:dbl)
                  n261 = Index Array(array=w281, index=w285) -> (element=w283:dbl)
                }
                n262 = for {
                  tunnel: w223 -> [w321] mode=indexing
                  tunnel: w207 -> [w320]
                  tunnel: [w318] -> w224 mode=indexing
                  tunnel: [w315] -> w225 mode=indexing
                  tunnel: w177 -> [w314]
                  tunnel: w191 -> [w313]
                  n263 = Search 1D Array(1D array=w320, element=w321) -> (index of element=w316:i32)  [unwired: 1 in]
                  n264 = Increment(x=w316) -> (x+1=w319:i32)
                  n265 = Increment(x=w316) -> (x+1=w317:i32)
                  n266 = Index Array(array=w314, index=w319) -> (element=w318:dbl)
                  n267 = Index Array(array=w313, index=w317) -> (element=w315:dbl)
                }
                n268 = property on="momentum graph" class="XYGraph (strict)"() -> ("Cursor.Cursor X"=w253:dbl)  [unwired: 2 in, 2 out]
                n269 = Search 1D Array(1D array=w177, element=w253) -> (index of element=w182:i32)  [unwired: 1 in]
                n270 = Index Array(array=w190, index (row)=w182) -> (element=→"Score":dbl[])  [unwired: 1 in]
                n271 = Array Max & Min(array=w177) -> (max value=w186:dbl)  [unwired: 3 out]
                n272 = Bundle(w177, w191) -> (w239:cluster{dbl[], dbl[]})  [unwired: 1 in]
                n273 = Bundle(w202, w201) -> (w197:cluster{dbl[], dbl[]})  [unwired: 1 in]
                n274 = Bundle(w177, w192) -> (w240:cluster{dbl[], dbl[]})  [unwired: 1 in]
                n275 = Bundle(w224, w225) -> (w199:cluster{dbl[], dbl[]})  [unwired: 1 in]
                n276 = Bundle(w204, w203) -> (w198:cluster{dbl[], dbl[]})  [unwired: 1 in]
                n277 = Decrement(x=w182) -> (x-1=w183:i32)
                n278 = Bundle(w219, w220) -> (w200:cluster{dbl[], dbl[]})  [unwired: 1 in]
                n279 = Delete From Array(array=w177, index=0) -> (array with subset deleted=w176:dbl[])  [unwired: 1 in, 1 out]
                n280 = Array Size(array=w190) -> (size(s)=w189:i32[])
                n281 = Index Array(array=w177, index #1=w182, index #2=w183) -> (element #1=w180:dbl, element #2=w181:dbl)
                n282 = Index Array(array=w189, index=0) -> (element=w187:i32)
                n283 = Subtract(x=w176, y=w177) -> (x-y=w175:dbl[])
                n284 = Build Array(w200, w199, w198, w197, w240, w239) -> (→"momentum graph":cluster{dbl[], dbl[]}[])
                n285 = Subtract(x=w180, y=w181) -> (x-y=→"Rally length(sec)":dbl)
                n286 = local read "edit video"() -> (w255:bool)
                n287 = Decrement(x=w187) -> (x-1=w185:i32)
                n288 = Divide(x=w186, y=w185) -> (x/y=→"Average rally length(sec)":dbl)
                n289 = Array Max & Min(array=w175) -> (max value=→"Longest rally length(sec)":dbl, min value=→"Shortest rally length(sec)":dbl)  [unwired: 2 out]
              }
              frame True {
                w423 = 0.0 ("Scale.Range:Minimum")
                # "used to sortout the frames service to point and editout the rest"
                n290 = call-poly <vilib>:"Read From Spreadsheet File.vi"("file path (dialog if empty)"="Data file") -> ("all rows"=w441:dbl[][])  [unwired: 6 in, 4 out]
                n291 = Delete From Array(array=w441, length=4, index (row)=0) -> (array with subset deleted=w420:dbl[][])  [unwired: 1 in, 1 out]
                "filedata in" <- w420
                n292 = Delete From Array(array=w420, length=2, index (col)=37 ("disabled index (col)")) -> (deleted portion=w432:dbl[][], array with subset deleted=w388:dbl[][])  [unwired: 1 in]
                "Score" <- w432
                n293 = Array Size(array=w432) -> (size(s)=w433:i32[])
                n294 = Index Array(array=w388, index (col) #1=31 ("disabled index (col)"), index (col) #2=32 ("index (col)"), index (col) #3=33 ("index (col)"), index (col) #4=34 ("index (col)")) -> (element #1=w415:dbl[], element #2=w414:dbl[], element #3=w413:dbl[], element #4=w412:dbl[])  [unwired: 4 in]
                n295 = Index Array(array=w433, index=0) -> (element=w431:i32)
                n296 = Or(x=w413, y=w412) -> (x .or. y?=w406:i32[])
                n297 = Or(x=w415, y=w414) -> (x .or. y?=w411:i32[])
                n298 = property on="Search score" class="Slide (strict)"("Scale.Maximum"=w431, "Scale.Minimum"=0.0 ("Scale.Range:Minimum")) -> ()  [unwired: 2 in, 2 out]
                n299 = Replace Array Subset(array=w388, new element #1=w411, index (col) #1=31 ("disabled index (col)"), new element #2=w411, index (col) #2=32 ("index (col)"), new element #3=w406, index (col) #3=33 ("index (col)"), new element #4=w406, index (col) #4=34 ("index (col)")) -> (w387:dbl[][])  [unwired: 4 in]
                n300 = Delete From Array(array=w387, length=1, index (col)=0 ("disabled index (col)")) -> (deleted portion=w435:dbl[][], array with subset deleted=w436:dbl[][])  [unwired: 1 in]
                n301 = case shown="True" "Playback\nscore" {
                  tunnel: w436 -> [w632 w639]
                  tunnel: w435 -> [w631 w638]
                  tunnel: w432 -> [_ w648]
                  tunnel: [w633 FALSE ("element")] -> w429
                  tunnel: [w631 w636] -> w386
                  tunnel: [w632 w635] -> w392
                  frame False {
                    n302 = local read "Playback\nscore"() -> (w633:bool)
                  }
                  frame True {
                    # "used to sort out the if the user asks for playback from score"
                    n303 = Index Array(array=w648, index (col) #1=0 ("disabled index (col)"), index (col) #2=1 ("index (col)")) -> (element #1=w645:dbl[], element #2=w644:dbl[])  [unwired: 2 in]
                    n304 = for {
                      tunnel: w645 -> [w668] mode=indexing
                      tunnel: w644 -> [w666] mode=indexing
                      tunnel: "P1 score" -> [w667]
                      tunnel: "P2 score" -> [w665]
                      tunnel: [w663] -> w640 mode=indexing
                      i -> [w662]
                      n305 = Equal?(x=w667, y=w668) -> (x = y?=w664:bool)
                      n306 = Equal?(x=w666, y=w665) -> (x = y?=w660:bool)
                      n307 = Increment(x=w662) -> (x+1=→"Search score":i32)
                      n308 = And(x=w664, y=w660) -> (x .and. y?=w663:bool)
                    }
                    n309 = property on="Search score" class="Slide (strict)"("Visible"=TRUE) -> ()  [unwired: 2 in, 2 out]
                    n310 = Or Array Elements(Boolean array=w640) -> (logical OR=w641:bool)
                    n311 = case shown="False" w641 {
                      tunnel: w640 -> [_ w659]
                      tunnel: w639 -> [w651 w657]
                      tunnel: w638 -> [w650 w656]
                      tunnel: [w651 w655] -> w635
                      tunnel: [w650 w654] -> w636
                      frame False {
                        n312 = One Button Dialog(message="This score has not\nbeen coded") -> ()  [unwired: 1 in, 1 out]
                      }
                      frame True {
                        n313 = Search 1D Array(1D array=w659, element=TRUE) -> (index of element=w653:i32)  [unwired: 1 in]
                        n314 = Increment(x=w653) -> (x+1=w652:i32)
                        n315 = Array Subset(array=w656, index (row)=w652) -> (w654:dbl[][])  [unwired: 3 in]
                        n316 = Array Subset(array=w657, index (row)=w652) -> (w655:dbl[][])  [unwired: 3 in]
                      }
                    }
                  }
                }
                "frame data" <- w386
                "coded data" <- w392
                n317 = Index Array(array=w388, index (col) #1=35 ("disabled index (col)"), index (col) #2=36 ("index (col)"), index (col) #3=37 ("index (col)"), index (col) #4=38 ("index (col)"), index (col) #5=39 ("index (col)"), index (col) #6=40 ("index (col)"), index (col) #7=0 ("index (col)")) -> (element #1=w396:dbl[], element #2=w397:dbl[], element #3=w395:dbl[], element #4=w394:dbl[], element #5=w381:dbl[], element #6=w380:dbl[], element #7=w385:dbl[])  [unwired: 7 in]
                n318 = Compound Arithmetic op=OR(w395, w394, w381, w380) -> (w398:i32[])
                n319 = for {
                  tunnel: w396 -> [w448] mode=indexing
                  tunnel: w385 -> [w452] mode=indexing
                  tunnel: w398 -> [w446] mode=indexing
                  tunnel: w397 -> [w447] mode=indexing
                  shift-right: [w454] -> w393
                  shift-left: dbl[] [] -> [w451]
                  tunnel: [FALSE ("edit video")] -> w391
                  w453 = 1.0 ("x")
                  n320 = Equal?(x=w453, y=w446) -> (x = y?=w455:bool)
                  n321 = Equal?(x=w453, y=w447) -> (x = y?=w456:bool)
                  n322 = Equal?(x=w453, y=w448) -> (x = y?=w457:bool)
                  n323 = Compound Arithmetic op=OR(w457, w456, w455) -> (w449:bool)
                  n324 = Insert Into Array(array=w451, new element=w452) -> (w450:dbl[])  [unwired: 1 in]
                  n325 = Select(t=w450, s=w449, f=w451) -> (s? t:f=w454:dbl[])
                }
                "serve to point" <- w393
                n326 = case shown="True" w427 {
                  tunnel: w392 -> [_ w525]
                  tunnel: w389 -> [_ w516]
                  tunnel: w386 -> [w477 w513]
                  tunnel: [w480 w506] -> w404
                  tunnel: [FALSE ("Visible") w505] -> w403
                  tunnel: w393 -> [_ w503]
                  tunnel: w386 -> [_ w499]
                  frame False {
                    n327 = Delete From Array(array=w477, length=1, index (col)=0 ("disabled index (col)")) -> (deleted portion=w476:dbl[][])  [unwired: 1 in, 1 out]
                    n328 = Array Max & Min(array=w476) -> (max value=w478:dbl, min value=w479:dbl)  [unwired: 2 out]
                    n329 = Build Array(w479, w478) -> (w480:dbl[])
                    n330 = One Button Dialog(message="Editing complete") -> ()  [unwired: 1 in, 1 out]
                  }
                  frame True {
                    w504 = dbl[] []
                    w517 = dbl[][] []
                    n331 = Array Size(array=w516) -> (size(s)=w510:i32)
                    n332 = Array Size(array=w513) -> (size(s)=w514:i32[])
                    n333 = for {
                      tunnel: w516 -> [w624] mode=indexing
                      tunnel: w525 -> [w621]
                      shift-right: [w620] -> w524
                      shift-left: w517 -> [w619]
                      tunnel: [w616] -> w508
                      i -> [w618]
                      n334 = Equal?(x=i16 1, y=w624) -> (x = y?=w622:bool)
                      n335 = case shown="True" w622 {
                        tunnel: w618 -> [_ w630]
                        tunnel: w621 -> [_ w629]
                        tunnel: [w625 w627] -> w620
                        tunnel: w619 -> [w625 w626]
                        frame False {
                        }
                        frame True {
                          n336 = Index Array(array=w629, index (col)=w630) -> (element=w628:dbl[])  [unwired: 1 in]
                          n337 = Insert Into Array(array=w626, new element=w628) -> (w627:dbl[][])  [unwired: 2 in]
                        }
                      }
                      n338 = Add(x=w618, y=2) -> (x+y=w616:i32)
                      "Search events" <- w616
                    }
                    n339 = Index Array(array=w514, index=0) -> (element=w509:i32)
                    n340 = local read "winner"() -> (w489:bool)
                    n341 = local read "error"() -> (w490:bool)
                    n342 = local read "point 1"() -> (w491:bool)
                    n343 = local read "point 2"() -> (w492:bool)
                    n344 = Add(x=w509, y=w510) -> (x+y=w512:i32)
                    n345 = Compound Arithmetic op=OR(w489, w490, w491, w492) -> (w488:bool)
                    n346 = property on="Search events" class="Slide (strict)"("Scale.Maximum"=w512, "Scale.Minimum"=0.0 ("Scale.Range:Minimum"), "Visible"=TRUE) -> ()  [unwired: 2 in, 2 out]
                    n347 = And(x=w488, y="Rally") -> (x .and. y?=w487:bool)
                    n348 = Transpose 2D Array(2D array=w524) -> (transposed array=w520:dbl[][])
                    n349 = Array Size(array=w520) -> (size(s)=w523:i32[])
                    n350 = local read "Serve1"() -> (w486:bool)
                    n351 = local read "Serve2"() -> (w485:bool)
                    n352 = local read "Serve3"() -> (w484:bool)
                    n353 = local read "Serve4"() -> (w483:bool)
                    n354 = Index Array(array=w523, index=0) -> (element=w521:i32)
                    n355 = for {
                      N: w521 -> [_]
                      tunnel: w513 -> [w609] mode=indexing
                      shift-right: [w608] -> w502
                      shift-left: w517 -> [w610]
                      tunnel: w520 -> [w607]
                      tunnel: [w604] -> w519 mode=indexing
                      tunnel: w508 -> [w601]
                      i -> [w602]
                      n356 = Index Array(array=w607, index (row)=w602) -> (element=w606:dbl[])  [unwired: 1 in]
                      n357 = Array Max & Min(array=w606) -> (min value=w605:dbl)  [unwired: 3 out]
                      n358 = Add(x=w602, y=w601) -> (x+y=w603:i32)
                      n359 = Equal?(x=w605, y=1) -> (x = y?=w604:bool)
                      n360 = local write "Search events"(w603) -> ()
                      n361 = case shown="True" w604 {
                        tunnel: w610 -> [w612 w615]
                        tunnel: w609 -> [_ w614]
                        tunnel: [w612 w613] -> w608
                        frame False {
                        }
                        frame True {
                          n362 = Insert Into Array(array=w615, new element=w614) -> (w613:dbl[][])  [unwired: 2 in]
                        }
                      }
                    }
                    "edited\nevents" <- w502
                    n363 = Or Array Elements(Boolean array=w519) -> (logical OR=w518:bool)
                    n364 = case shown="False" w518 {
                      frame False {
                        n365 = One Button Dialog(message="This combination \nof events are \nnot available") -> ()  [unwired: 1 in, 1 out]
                      }
                      frame True {
                        n366 = One Button Dialog(message="Editing complete") -> ()  [unwired: 1 in, 1 out]
                      }
                    }
                    n367 = Compound Arithmetic op=OR(w486, w485, w484, w483) -> (w496:bool)
                    n368 = And(x=w496, y="3 shots") -> (x .and. y?=w494:bool)
                    n369 = Build Array(w487, w494) -> (w498:bool[])
                    n370 = Index Array(array=w502, index (col)=0 ("disabled index (col)")) -> (element=w500:dbl[])  [unwired: 1 in]
                    n371 = Boolean Array To Number(Boolean array=w498) -> (number=w497:u32)
                    n372 = case shown="0, Default" w497 {
                      tunnel: w502 -> [w529 _ _]
                      tunnel: [w528 w563 w579] -> w506
                      tunnel: [w527 FALSE ("Visible") FALSE ("Visible")] -> w505
                      tunnel: w504 -> [w526 _ _]
                      tunnel: w504 -> [_ w565 w583]
                      tunnel: w503 -> [_ w564 _]
                      tunnel: w500 -> [_ w561 w584]
                      tunnel: w499 -> [_ _ w582]
                      frame 0, Default {
                        n373 = Index Array(array=w529, index (col)=0 ("disabled index (col)")) -> (element=w531:dbl[])  [unwired: 1 in]
                        n374 = Array Size(array=w529) -> (size(s)=w535:i32[])
                        n375 = Multiply(x="after", y=25.0) -> (x*y=w533:dbl)
                        n376 = Index Array(array=w535, index=0) -> (element=w530:i32)
                        n377 = Multiply(x="before", y=25.0) -> (x*y=w534:dbl)
                        n378 = for {
                          N: w530 -> [_]
                          tunnel: w534 -> [w551]
                          tunnel: w533 -> [w553]
                          tunnel: w531 -> [w552] mode=indexing
                          shift-right: [w543] -> w528
                          shift-left: w526 -> [w547]
                          tunnel: [FALSE ("Visible")] -> w527
                          n379 = Subtract(x=w552, y=w551) -> (x-y=w549:dbl)
                          n380 = Add(x=w553, y=w552) -> (x+y=w548:dbl)
                          n381 = Array Max & Min(array=w547) -> (max value=w550:dbl, max index (indices)=w545:i32)  [unwired: 2 out]
                          n382 = Greater Or Equal?(x=w550, y=w549) -> (x >= y?=w546:bool)
                          n383 = Build Array(w549, w548) -> (w542:dbl[])
                          n384 = Build Array(w548) -> (w544:dbl[])
                          n385 = case shown="True" w546 {
                            tunnel: w547 -> [w556 w560]
                            tunnel: w545 -> [_ w559]
                            tunnel: w544 -> [_ w558]
                            tunnel: [w555 w557] -> w543
                            tunnel: w542 -> [w554 _]
                            frame False {
                              n386 = Insert Into Array(array=w556, new element=w554) -> (w555:dbl[])  [unwired: 1 in]
                            }
                            frame True {
                              n387 = Replace Array Subset(array=w560, new element=w558, index=w559) -> (w557:dbl[])
                            }
                          }
                        }
                      }
                      frame 1 {
                        n388 = for {
                          tunnel: w561 -> [w566] mode=indexing
                          shift-right: [w573] -> w563
                          shift-left: w565 -> [w574]
                          tunnel: w564 -> [w567]
                          n389 = Search 1D Array(1D array=w567, element=w566) -> (index of element=w578:i32)  [unwired: 1 in]
                          n390 = Add(x=50.0, y=w566) -> (x+y=w571:dbl)
                          n391 = Subtract(x=w578, y=1) -> (x-y=w576:i32)
                          n392 = Index Array(array=w567, index=w576) -> (element=w568:dbl)
                          n393 = Subtract(x=w568, y=50.0 ("x")) -> (x-y=w572:dbl)
                          n394 = Build Array(w572, w571) -> (w575:dbl[])
                          n395 = Insert Into Array(array=w574, new element=w575) -> (w573:dbl[])  [unwired: 1 in]
                        }
                      }
                      frame 2 {
                        n396 = Index Array(array=w582, index (col)=0 ("disabled index (col)")) -> (element=w580:dbl[])  [unwired: 1 in]
                        n397 = for {
                          tunnel: w584 -> [w588] mode=indexing
                          shift-right: [w596] -> w579
                          shift-left: w583 -> [w597]
                          tunnel: w580 -> [w591]
                          n398 = Search 1D Array(1D array=w591, element=w588) -> (index of element=w590:i32)  [unwired: 1 in]
                          n399 = Add(x=w590, y="shots") -> (x+y=w589:i32)
                          n400 = Subtract(x=w588, y=50.0 ("x")) -> (x-y=w595:dbl)
                          n401 = Index Array(array=w591, index=w589) -> (element=w587:dbl)
                          n402 = Add(x=25.0, y=w587) -> (x+y=w594:dbl)
                          n403 = Build Array(w595, w594) -> (w598:dbl[])
                          n404 = Insert Into Array(array=w597, new element=w598) -> (w596:dbl[])  [unwired: 1 in]
                        }
                      }
                    }
                  }
                }
                "edited to play" <- w404
                n405 = local write "Playback\nscore"(w429) -> ()
                n406 = property on="Search score" class="Slide (strict)"("Visible"=w429) -> ()  [unwired: 2 in, 2 out]
                n407 = Array Size(array=w404) -> (size(s)=w426:i32)
                n408 = property on="Search events" class="Slide (strict)"("Visible"=w403) -> ()  [unwired: 2 in, 2 out]
                n409 = Divide(x=w426, y=2) -> (x/y=w422:dbl)
                n410 = for {
                  N: w422 -> [_]
                  shift-right: [w462] -> _
                  shift-left: w404 -> [w464]
                  tunnel: [w458] -> w424
                  n411 = Split 1D Array(array=w464, index=2) -> (first subarray=w463:dbl[], second subarray=w462:dbl[])
                  n412 = Index Array(array=w463, index #1=1 ("index"), index #2=0 ("index")) -> (element #1=w468:dbl, element #2=w461:dbl)
                  n413 = Subtract(x=w468, y=w461) -> (x-y=w460:dbl)
                  n414 = Increment(x=w460) -> (x+1=w459:dbl)
                  n415 = for {
                    N: w459 -> [_]
                    tunnel: w461 -> [w473]
                    tunnel: [w469] -> w458
                    i -> [w472]
                    n416 = local read "frames"() -> (w471:dbl[])
                    n417 = Add(x=w473, y=w472) -> (x+y=w470:dbl)
                    n418 = Insert Into Array(array=w471, new element=w470) -> (w469:dbl[])  [unwired: 1 in]
                    n419 = local write "frames"(w469) -> ()
                  }
                }
                n420 = Array Size(array=w424) -> (size(s)=w421:i32)
                n421 = property on="play back" class="Slide (strict)"("Scale.Maximum"=w421, "Scale.Minimum"=w423, "Maximum"=w421) -> ()  [unwired: 2 in, 2 out]
                n422 = property on="writing" class="Slide (strict)"("Scale.Maximum"=w421, "Scale.Minimum"=w423) -> ()  [unwired: 2 in, 2 out]
                "frames" <- w425
              }
            }
            n423 = local write "edit video"(w159) -> ()
          }
          frame #1 {
            w774 = 0.0 ("X Scale.Range:Minimum")
            w811 = i16 1 ("width (-)")
            w938 = dbl[] [0.0, 0.0, 0.0, 0.0, 0.0, 0.0, 0.0, 0.0, 0.0, 0.0, 0.0] ("array")
            w926 = string[] ["Winners", "Errors"] ("W/E1")
            w907 = string[] ["Fore hand", "Back hand", "Over head", "", "Straight", "Cross", "", "Smash", "Half smash", "DRIVE DEF", "BLOCK DEF", "CLEAR DEF", "Drive/Tap", "Lob", "Drop", "Clear", "Net"] ("Player 2")
            w901 = "" ("new element/subarray")
            w900 = "" ("new element/subarray")
            w865 = 15 ("index")
            w860 = 15 ("index")
            # "seperate player 1 n 2 data"
            n424 = local read "edited\nevents"() -> (w831:dbl[][])
            n425 = local read "Compare"() -> (w788:bool)
            n426 = local read "filedata in"() -> (w837:dbl[][])
            n427 = Array Size(array=w831) -> (size(s)=w843:i32[])
            n428 = case shown="False" w788 {
              frame False {
                w939 = u8 0 ("Disabled")
                n429 = local read "Percentage"() -> (w940:bool)
                n430 = local write "Percentage"(w940) -> ()
                n431 = local read "display\nselection"() -> (w941:string)
                n432 = local write "display\nselection"(w941) -> ()
                n433 = property on="display\nselection" class="CmbBox"("Disabled"=w939) -> ()  [unwired: 2 in, 2 out]
                n434 = property on="Percentage" class="Bool (strict)"("Disabled"=w939) -> ()  [unwired: 2 in, 2 out]
              }
              frame True {
                w942 = u8 2 ("Disabled")
                n435 = local read "1"() -> (w944:string)
                n436 = local write "display\nselection"(w944) -> ()
                n437 = property on="display\nselection" class="CmbBox"("Disabled"=w942) -> ()  [unwired: 2 in, 2 out]
                n438 = property on="Percentage" class="Bool (strict)"("Disabled"=w942) -> ()  [unwired: 2 in, 2 out]
                n439 = local write "Percentage"(TRUE ("t")) -> ()
              }
            }
            n440 = Index Array(array=w837, index (col)=0 ("disabled index (col)")) -> (element=w839:dbl[])  [unwired: 1 in]
            n441 = Index Array(array=w831, index (col)=0 ("disabled index (col)")) -> (element=w836:dbl[])  [unwired: 1 in]
            n442 = Index Array(array=w843, index=0) -> (element=w841:i32)
            n443 = local read "comp_p1 2"() -> (w786:dbl[])
            n444 = local read "Compare"() -> (w795:bool)
            n445 = for {
              N: w841 -> [_]
              tunnel: w839 -> [w966]
              tunnel: w836 -> [w965] mode=indexing
              tunnel: [w962] -> w830 mode=indexing
              i -> [w967]
              n446 = Search 1D Array(1D array=w966, element=w965, start index (0)=w967) -> (index of element=w963:i32)
              n447 = local read "filedata in"() -> (w964:dbl[][])
              n448 = Index Array(array=w964, index (row)=w963) -> (element=w962:dbl[])  [unwired: 1 in]
            }
            n449 = case shown="\"2\"" "display\nselection" {
              tunnel: [w952 w953 w954 w955] -> w746
              tunnel: w830 -> [_ w953 _ _]
              frame "1", Default {
                n450 = local read "filedata in"() -> (w952:dbl[][])
              }
              frame "2" {
              }
              frame "3" {
                n451 = local read "save1_data"() -> (w954:dbl[][])
              }
              frame "4" {
                n452 = local read "save2_data"() -> (w955:dbl[][])
              }
            }
            n453 = Index Array(array=w746, index (col) #1=31 ("disabled index (col)"), index (col) #2=33 ("index (col)"), index (col) #3=32 ("index (col)"), index (col) #4=34 ("index (col)")) -> (element #1=w909:dbl[], element #2=w914:dbl[], element #3=w915:dbl[], element #4=w913:dbl[])  [unwired: 4 in]
            n454 = Index Array(array=w746, index (col) #1=48 ("disabled index (col)"), index (col) #2=49 ("index (col)")) -> (element #1=w850:dbl[], element #2=w847:dbl[])  [unwired: 2 in]
            n455 = Add Array Elements(numeric array=w909) -> (sum=w929:dbl)
            n456 = Add Array Elements(numeric array=w915) -> (sum=w928:dbl)
            n457 = local read "Compare"() -> (w798:bool)
            n458 = Add Array Elements(numeric array=w913) -> (sum=w927:dbl)
            n459 = Add Array Elements(numeric array=w914) -> (sum=w930:dbl)
            n460 = local read "comp_p2 2"() -> (w794:dbl[])
            n461 = local read "Percentage"() -> (w905:bool)
            n462 = Build Array(w929, w930) -> (w797:dbl[])
            n463 = Build Array(w928, w927) -> (w787:dbl[])
            n464 = for {
              N: 38 -> [_]
              tunnel: w746 -> [w1002]
              tunnel: w850 -> [w1001]
              tunnel: w847 -> [w1000]
              tunnel: [w998] -> w848 mode=indexing
              tunnel: [w997] -> w849 mode=indexing
              i -> [w995]
              n465 = Increment(x=w995) -> (x+1=w996:i32)
              n466 = Index Array(array=w1002, index (col)=w996) -> (element=w999:dbl[])  [unwired: 1 in]
              n467 = And(x=w1001, y=w999) -> (x .and. y?=w998:i32[])
              n468 = And(x=w1000, y=w999) -> (x .and. y?=w997:i32[])
            }
            n469 = Select(t=w794, s=w795, f=w787) -> (s? t:f=w793:dbl[])
            n470 = Select(t=w786, s=w798, f=w797) -> (s? t:f=w796:dbl[])
            n471 = local read "Percentage"() -> (w906:bool)
            n472 = Number To Decimal String(number=w796, width (-)=w811) -> (decimal integer string=→"W1/E1":string[])
            n473 = Number To Decimal String(number=w793, width (-)=w811) -> (decimal integer string=→"W2/E2":string[])
            n474 = Transpose 2D Array(2D array=w848) -> (transposed array=w859:i32[][])
            n475 = Transpose 2D Array(2D array=w849) -> (transposed array=w858:i32[][])
            n476 = for {
              N: 30 -> [_]
              tunnel: w859 -> [w994]
              tunnel: w858 -> [w993]
              tunnel: [w990] -> w758 mode=indexing
              tunnel: [w989] -> w765 mode=indexing
              i -> [w992]
              # "adds the data"
              n477 = Index Array(array=w994, index (col)=w992) -> (element=w991:i32[])  [unwired: 1 in]
              n478 = Index Array(array=w993, index (col)=w992) -> (element=w988:i32[])  [unwired: 1 in]
              n479 = Add Array Elements(numeric array=w991) -> (sum=w990:i32)
              n480 = Add Array Elements(numeric array=w988) -> (sum=w989:i32)
            }
            n481 = Number To Fractional String(number=w765, precision (6)=i16 0) -> (F-format string=w764:string[])  [unwired: 2 in]
            n482 = Number To Fractional String(number=w758, precision (6)=i16 0) -> (F-format string=w760:string[])  [unwired: 2 in]
            n483 = Insert Into Array(array=w758, new element=w786) -> (w835:i32[])  [unwired: 1 in]
            n484 = Insert Into Array(array=w765, new element=w787) -> (w834:i32[])  [unwired: 1 in]
            n485 = Build Array(w835, w834) -> (w828:i32[][])
            n486 = case shown="\"0\", Default" "display\nselection" {
              tunnel: w828 -> [_ w951 _]
              frame "0", Default {
              }
              frame "1" {
                "game" <- w951
              }
              frame "2" {
              }
            }
            n487 = case shown="True" "save2" {
              tunnel: w828 -> [_ w958]
              tunnel: w746 -> [_ w956]
              frame False {
              }
              frame True {
                n488 = local write "save2"(FALSE ("save2")) -> ()
                "save2" <- w958
                "save2_data" <- w956
              }
            }
            n489 = case shown="True" "save1" {
              tunnel: w828 -> [_ w961]
              tunnel: w746 -> [_ w959]
              frame False {
              }
              frame True {
                n490 = local write "save1"(FALSE ("save1")) -> ()
                "save1" <- w961
                "save1_data" <- w959
              }
            }
            n491 = Split 1D Array(array=w765, index=15) -> (second subarray=w891:i32[])  [unwired: 1 out]
            n492 = Split 1D Array(array=w758, index=w860) -> (first subarray=w861:i32[], second subarray=w870:i32[])
            n493 = Split 1D Array(array=w765, index=w865) -> (first subarray=w864:i32[], second subarray=w869:i32[])
            n494 = Split 1D Array(array=w758, index=15) -> (second subarray=w885:i32[])  [unwired: 1 out]
            n495 = local read "Percentage"() -> (w895:bool)
            n496 = Add Array Elements(numeric array=w861) -> (sum=w862:i32)
            n497 = Add Array Elements(numeric array=w864) -> (sum=w863:i32)
            n498 = Number To Decimal String(number=w891, width (-)=i16 1 ("precision (6)")) -> (decimal integer string=w743:string[])
            n499 = Number To Decimal String(number=w885, width (-)=i16 1 ("precision (6)")) -> (decimal integer string=w894:string[])
            n500 = for {
              N: w860 -> [_]
              tunnel: w861 -> [w987] mode=indexing
              tunnel: w862 -> [w986]
              tunnel: [w983] -> w880 mode=indexing
              n501 = Divide(x=w987, y=w986) -> (x/y=w985:dbl)
              n502 = Multiply(x=w985, y=100.0) -> (x*y=w983:dbl)
            }
            n503 = Index Array(array=w870, index #1=3 ("index"), index #2=4 ("index")) -> (element #1=w866:i32, element #2=w867:i32)
            n504 = for {
              N: w865 -> [_]
              tunnel: w864 -> [w982] mode=indexing
              tunnel: w863 -> [w981]
              tunnel: [w978] -> w790 mode=indexing
              n505 = Divide(x=w982, y=w981) -> (x/y=w980:dbl)
              n506 = Multiply(x=w980, y=100.0) -> (x*y=w978:dbl)
            }
            n507 = Index Array(array=w869, index #1=3 ("index"), index #2=4 ("index")) -> (element #1=w857:i32, element #2=w856:i32)
            n508 = case shown="\"1\", Default" "2" {
              tunnel: [w945 w946 w947] -> w820
              frame "1", Default {
                n509 = local read "game"() -> (w945:i32[][])
              }
              frame "3" {
                n510 = local read "save1"() -> (w946:i32[][])
              }
              frame "4" {
                n511 = local read "save2"() -> (w947:i32[][])
              }
            }
            n512 = Add(x=w866, y=w867) -> (x+y=w742:i32)
            n513 = case shown="\"1\", Default" "1" {
              tunnel: [w948 w949 w950] -> w824
              frame "1", Default {
                n514 = local read "game"() -> (w948:i32[][])
              }
              frame "3" {
                n515 = local read "save1"() -> (w949:i32[][])
              }
              frame "4" {
                n516 = local read "save2"() -> (w950:i32[][])
              }
            }
            n517 = Add(x=w857, y=w856) -> (x+y=w868:i32)
            n518 = for {
              tunnel: w870 -> [w972] mode=indexing
              tunnel: w742 -> [w971]
              tunnel: [w968] -> w881 mode=indexing
              n519 = Divide(x=w972, y=w971) -> (x/y=w970:dbl)
              n520 = Multiply(x=w970, y=100.0) -> (x*y=w968:dbl)
            }
            n521 = for {
              tunnel: w869 -> [w977] mode=indexing
              tunnel: w868 -> [w976]
              tunnel: [w973] -> w882 mode=indexing
              n522 = Divide(x=w977, y=w976) -> (x/y=w975:dbl)
              n523 = Multiply(x=w975, y=100.0) -> (x*y=w973:dbl)
            }
            n524 = local read "Compare"() -> (w801:bool)
            n525 = local read "comp_p2"() -> (w802:dbl[])
            n526 = local read "comp_p1"() -> (w803:dbl[])
            n527 = Index Array(array=w820, index (row) #1=0 ("index (row)"), index (row) #2=1 ("index (row)")) -> (element #1=w818:i32[], element #2=w816:i32[])  [unwired: 2 in]
            n528 = Index Array(array=w824, index (row) #1=0 ("index (row)"), index (row) #2=1 ("index (row)")) -> (element #1=w819:i32[], element #2=w817:i32[])  [unwired: 2 in]
            n529 = Insert Into Array(array=w880, new element=w881) -> (w791:dbl[])  [unwired: 1 in]
            n530 = Insert Into Array(array=w790, new element=w882) -> (w789:dbl[])  [unwired: 1 in]
            n531 = Divide(x=w819, y=w818) -> (x/y=w813:dbl[])
            n532 = Divide(x=w817, y=w816) -> (x/y=w812:dbl[])
            n533 = Select(t=w803, s="Compare", f=w791) -> (s? t:f=w762:dbl[])
            n534 = Number To Fractional String(number=w762, precision (6)=i16 0) -> (F-format string=w759:string[])  [unwired: 2 in]
            n535 = Select(t=w759, s=w906, f=w760) -> (s? t:f=w748:string[])
            n536 = call "Search NaN_Inf (SubVI).vi"("in"=w748) -> ("out"=w747:string[])
            n537 = Index Array(array=w747, index #1=0 ("index"), index #2=1 ("index"), index #3=2 ("index"), index #4=3 ("index"), index #5=4 ("index"), index #6=5 ("index"), index #7=6 ("index"), index #8=7 ("index"), index #9=8 ("index"), index #10=9 ("index"), index #11=10 ("index"), index #12=11 ("index"), index #13=12 ("index"), index #14=13 ("index"), index #15=14 ("index")) -> (element #1=→"p1 1":string, element #2=→"p1 2":string, element #3=→"p1 3":string, element #4=→"p1 4":string, element #5=→"p1 5":string, element #6=→"p1 6":string, element #7=→"p1 7":string, element #8=→"p1 8":string, element #9=→"p1 9":string, element #10=→"p1 10":string, element #11=→"p1 11":string, element #12=→"p1 12":string, element #13=→"p1 13":string, element #14=→"p1 14":string, element #15=→"p1 15":string)
            n538 = Split 1D Array(array=w762, index=15) -> (second subarray=w887:dbl[])  [unwired: 1 out]
            n539 = Number To Fractional String(number=w887, precision (6)=i16 0) -> (F-format string=w893:string[])  [unwired: 2 in]
            n540 = Select(t=w893, s="Percentage", f=w894) -> (s? t:f=w740:string[])
            n541 = call "Search NaN_Inf (SubVI).vi"("in"=w740) -> ("out"=w773:string[])
            n542 = Insert Into Array(array=w773, index=3, new element=w900) -> (w898:string[])
            n543 = Insert Into Array(array=w898, index=6, new element=w900) -> (w916:string[])
            n544 = Split 1D Array(array=w916, index=6) -> (first subarray=→"player1_2":string[], second subarray=w919:string[])
            n545 = Select(t=w802, s=w801, f=w789) -> (s? t:f=w768:dbl[])
            n546 = Number To Fractional String(number=w768, precision (6)=i16 0) -> (F-format string=w767:string[])  [unwired: 2 in]
            n547 = Select(t=w767, s=w905, f=w764) -> (s? t:f=w769:string[])
            n548 = call "Search NaN_Inf (SubVI).vi"("in"=w769) -> ("out"=w710:string[])
            n549 = Index Array(array=w710, index #1=0 ("index"), index #2=1 ("index"), index #3=2 ("index"), index #4=3 ("index"), index #5=4 ("index"), index #6=5 ("index"), index #7=6 ("index"), index #8=7 ("index"), index #9=8 ("index"), index #10=9 ("index"), index #11=10 ("index"), index #12=11 ("index"), index #13=12 ("index"), index #14=13 ("index"), index #15=14 ("index")) -> (element #1=→"p2 17":string, element #2=→"p2 16":string, element #3=→"p2 12":string, element #4=→"p2 13":string, element #5=→"p2 15":string, element #6=→"p2 14":string, element #7=→"p2 10":string, element #8=→"p2 11":string, element #9=→"p2 9":string, element #10=→"p2 18":string, element #11=→"p2 19":string, element #12=→"p2 20":string, element #13=→"p2 21":string, element #14=→"p2 22":string, element #15=→"p2 23":string)
            n550 = Split 1D Array(array=w768, index=15) -> (second subarray=w888:dbl[])  [unwired: 1 out]
            n551 = Number To Fractional String(number=w888, precision (6)=i16 0) -> (F-format string=w744:string[])  [unwired: 2 in]
            n552 = Select(t=w744, s=w895, f=w743) -> (s? t:f=w741:string[])
            n553 = call "Search NaN_Inf (SubVI).vi"("in"=w741) -> ("out"=w745:string[])
            n554 = Insert Into Array(array=w745, index=3, new element=w901) -> (w903:string[])
            n555 = Insert Into Array(array=w903, index=6, new element=w901) -> (w924:string[])
            n556 = Split 1D Array(array=w924, index=6) -> (first subarray=→"player2_2":string[], second subarray=w922:string[])
            n557 = Multiply(x=w812, y=100.0 ("new element/subarray")) -> (x*y=w807:dbl[])
            n558 = Delete From Array(array=w919, index=0) -> (array with subset deleted=w671:string[])  [unwired: 1 in, 1 out]
            n559 = Multiply(x=100.0 ("new element/subarray"), y=w813) -> (x*y=w810:dbl[])
            n560 = Delete From Array(array=w922, index=0) -> (array with subset deleted=w683:string[])  [unwired: 1 in, 1 out]
            n561 = Split 1D Array(array=w810, index=30) -> (first subarray=→"comp_p1":dbl[], second subarray=→"comp_p1 2":dbl[])
            n562 = Split 1D Array(array=w807, index=30) -> (first subarray=→"comp_p2":dbl[], second subarray=→"comp_p2 2":dbl[])
            n563 = Delete From Array(array=w671, length=2, index=8) -> (deleted portion=w681:string[], array with subset deleted=w672:string[])
            n564 = Delete From Array(array=w683, length=2, index=8) -> (deleted portion=w685:string[], array with subset deleted=w694:string[])
            n565 = Delete From Array(array=w672, length=1, index=5) -> (deleted portion=w678:string[], array with subset deleted=w677:string[])
            n566 = Delete From Array(array=w694, length=1, index=5) -> (deleted portion=w688:string[], array with subset deleted=w689:string[])
            n567 = Insert Into Array(array=w677, index=1, new element=w678) -> (w680:string[])
            n568 = Insert Into Array(array=w689, index=1, new element=w688) -> (w686:string[])
            n569 = Insert Into Array(array=w680, index=3, new element=w681) -> (w670:string[])
            "player1 2" <- w670
            n570 = Fract/Exp String To Number(string=w670) -> (number=w772:dbl[])  [unwired: 3 in, 1 out]
            n571 = Interleave 1D Arrays(w938, w772) -> (w785:dbl[])
            n572 = Array Max & Min(array=w772) -> (max value=w782:dbl)  [unwired: 3 out]
            n573 = Insert Into Array(array=w785, new element=0.0 ("new element/subarray")) -> (w934:dbl[])  [unwired: 1 in]
            n574 = Bundle(w934, "array"=dbl[] [1.0, 2.0, 3.0, 4.0, 5.0, 6.0, 7.0, 8.0, 9.0, 10.0, 11.0, 12.0, 13.0, 14.0, 15.0, 16.0, 17.0, 18.0, 19.0, 20.0, 21.0]) -> (→"P1graph":cluster{dbl[], "array":dbl[]})  [unwired: 1 in]
            n575 = Insert Into Array(array=w686, index=3, new element=w685) -> (w669:string[])
            "player2 2" <- w669
            n576 = Fract/Exp String To Number(string=w669) -> (number=w771:dbl[])  [unwired: 3 in, 1 out]
            n577 = Array Max & Min(array=w771) -> (max value=w781:dbl)  [unwired: 3 out]
            n578 = Interleave 1D Arrays(w938, w771) -> (w783:dbl[])
            n579 = Insert Into Array(array=w783, new element=0.0 ("new element/subarray")) -> (w935:dbl[])  [unwired: 1 in]
            n580 = Max & Min(x=w782, y=w781) -> (max(x,y)=w776:dbl)  [unwired: 1 out]
            n581 = Bundle(w935, "array"=dbl[] [1.0, 2.0, 3.0, 4.0, 5.0, 6.0, 7.0, 8.0, 9.0, 10.0, 11.0, 12.0, 13.0, 14.0, 15.0, 16.0, 17.0, 18.0, 19.0, 20.0, 21.0]) -> (→"P2graph":cluster{dbl[], "array":dbl[]})  [unwired: 1 in]
            n582 = Equal?(x=w776, y=inf) -> (x = y?=w778:bool)
            n583 = Select(t=100.0, s=w778, f=w776) -> (s? t:f=w775:dbl)
            n584 = property on="P2graph" class="XYGraph (strict)"("XScale.Maximum"=w775, "XScale.Minimum"=w774) -> ()  [unwired: 2 in, 2 out]
            n585 = property on="P1graph" class="XYGraph (strict)"("XScale.Maximum"=w775, "XScale.Minimum"=w774) -> ()  [unwired: 2 in, 2 out]
            "Player 1" <- w907
            "Player 1_2" <- w907
            "Player 2_2" <- w907
            "Player 2" <- w907
            "W/E1" <- w926
            "W/E2" <- w926
          }
        }
        n586 = case shown="True" "Play" {
          frame False {
            w1003 = 0 ("play back")
            n587 = property on="Compare" class="Bool (strict)"("DisabledEnum"=w1003) -> ()  [unwired: 2 in, 2 out]
            n588 = property on="Percentage" class="Bool (strict)"("DisabledEnum"=w1003) -> ()  [unwired: 2 in, 2 out]
            n589 = property on="save1" class="Bool (strict)"("DisabledEnum"=w1003) -> ()  [unwired: 2 in, 2 out]
            n590 = property on="save2" class="Bool (strict)"("DisabledEnum"=w1003) -> ()  [unwired: 2 in, 2 out]
            n591 = property on="display\nselection" class="CmbBox"("DisabledEnum"=w1003) -> ()  [unwired: 2 in, 2 out]
          }
          frame True {
            w1016 = T4 4 items=["Grayscale (U8)", "Grayscale (I16)", "Grayscale (SGL)", "Complex (CSG)", "RGB (U32)", "HSL (U32)", "RGB (U64)"] ("Image Type")
            n592 = local read "Vid file"() -> (w1009:path)
            n593 = local write "play back"(0 ("play back")) -> ()
            n594 = local write "Play"(FALSE ("Play")) -> ()
            n595 = call "IMAQ AVI Open"("AVI Path"=w1009) -> ("error out"=w1006:errorcluster, "Avi Refnum"=w1008:T5)  [unwired: 9 in]
            n596 = call "IMAQ Create"("Image Name"="Disp1", "Image Type"=w1016) -> ("New Image"=w1015:T1, "error out"=w1014:errorcluster)  [unwired: 3 in]
            n597 = call "IMAQ AVI Get Info"("error in (no error)"=w1006, "Avi Refnum"=w1008) -> ("Avi Refnum (duplicate)"=w1007:T5, "Frame Data"=w1005:T6)  [unwired: 5 in, 3 out]
            n598 = Unbundle By Name(w1005) -> ("framesPerSecond"=w1004:u32)
            n599 = while {
              tunnel: w1007 -> [w1037]
              tunnel: w1015 -> [w1039]
              tunnel: w1014 -> [w1038]
              tunnel: [FALSE ("Play")] -> w1010
              tunnel: [w1019] -> w1012
              tunnel: w1004 -> [w1020]
              stop <- w1030 stop-if-true
              w1018 = 2 ("play back")
              n600 = local read "frames"() -> (w1035:dbl[])
              n601 = Increment(x="play back") -> (x+1=w1026:i32)
              n602 = Index Array(array=w1035, index=w1026) -> (element=w1034:dbl)
              n603 = Array Max & Min(array=w1035) -> (max value=w1033:dbl)  [unwired: 3 out]
              n604 = Divide(x=w1026, y=25.0) -> (x/y=→"Numeric":dbl)
              n605 = local write "play back"(w1026) -> ()
              n606 = Divide(x=1000.0, y="Playback Speed") -> (x/y=w1023:dbl)
              n607 = Divide(x=w1023, y=w1020) -> (x/y=w1024:dbl)
              n608 = Equal?(x=w1034, y=w1033) -> (x = y?=w1032:bool)
              n609 = call "IMAQ AVI Read Frame"("error in (no error)"=w1038, "Frame Number"=w1034, "Image"=w1039, "Avi Refnum"=w1037) -> ("Image Out"=→"DISP":T1, "Avi Refnum (duplicate)"=w1019:T5)  [unwired: 4 in, 2 out]
              n610 = Wait (ms)(milliseconds to wait=w1024) -> ()  [unwired: 1 out]
              n611 = Or(x=w1032, y="stop 2") -> (x .or. y?=w1030:bool)
              n612 = while {
                stop <- w1040 continue-if-true
                n613 = local read "stop 2"() -> (w1043:bool)
                n614 = Not(x=w1043) -> (.not. x?=w1042:bool)
                n615 = And(x=w1042, y="pause") -> (x .and. y?=w1040:bool)
              }
              n616 = property on="Compare" class="Bool (strict)"("DisabledEnum"=w1018) -> ()  [unwired: 2 in, 2 out]
              n617 = property on="Percentage" class="Bool (strict)"("DisabledEnum"=w1018) -> ()  [unwired: 2 in, 2 out]
              n618 = property on="save1" class="Bool (strict)"("DisabledEnum"=w1018) -> ()  [unwired: 2 in, 2 out]
              n619 = property on="save2" class="Bool (strict)"("DisabledEnum"=w1018) -> ()  [unwired: 2 in, 2 out]
              n620 = property on="display\nselection" class="CmbBox"("DisabledEnum"=w1018) -> ()  [unwired: 2 in, 2 out]
            }
            n621 = local write "stop 2"(w1010) -> ()
            n622 = call "IMAQ AVI Close"("Avi Refnum"=w1012) -> ()  [unwired: 10 in, 1 out]
          }
        }
        n623 = case shown="True" "write file" {
          frame False {
          }
          frame True {
            n624 = local write "writing"(0 ("writing")) -> ()
            n625 = call <vilib>:"Get File Extension.vi"("file"="Write VI") -> ("filename without extension"=w97:string)  [unwired: 7 in, 3 out]
            n626 = Strip Path(path="Write VI") -> (stripped path=w98:path)  [unwired: 1 out]
            n627 = call <vilib>:"Check if File or Folder Exists.vi"("path"=w98) -> ("file or folder exists?"=w99:bool)  [unwired: 8 in, 2 out]
            n628 = case shown="True" w99 {
              tunnel: w98 -> [_ w113]
              tunnel: w97 -> [_ w112]
              frame False {
                w100 = FALSE ("Visible")
                n629 = local write "Write VI"(path "" ("Write VI")) -> ()
                n630 = property on="writing" class="Slide (strict)"("Visible"=w100) -> ()  [unwired: 2 in, 2 out]
                n631 = local write "write file"(w100) -> ()
              }
              frame True {
                w127 = T4 4 items=["Grayscale (U8)", "Grayscale (I16)", "Grayscale (SGL)", "Complex (CSG)", "RGB (U32)", "HSL (U32)", "RGB (U64)"] ("Image Type")
                n632 = local read "Vid file"() -> (w106:path)
                n633 = Path To String(path=w113) -> (string=w115:string)
                n634 = property on="writing" class="Slide (strict)"("Visible"=TRUE) -> ()  [unwired: 2 in, 2 out]
                n635 = call "IMAQ AVI Open"("AVI Path"=w106) -> ("error out"=w109:errorcluster, "Avi Refnum"=w110:T5)  [unwired: 9 in]
                n636 = Concatenate Strings(w115, "\\" ("string"), w112, ".avi" ("string")) -> (w114:string)
                n637 = call "IMAQ AVI Get Info"("error in (no error)"=w109, "Avi Refnum"=w110) -> ("Avi Refnum (duplicate)"=w111:T5, "Frame Data"=w108:T6)  [unwired: 5 in, 3 out]
                n638 = Unbundle By Name(w108) -> ("framesPerSecond"=w107:u32)
                n639 = String To Path(string=w114) -> (path=w104:path)
                n640 = local write "Write VI"(w104) -> ()
                n641 = local read "frames"() -> (w105:dbl[])
                n642 = call "IMAQ Create"("Image Name"="write", "Image Type"=w127) -> ("New Image"=w125:T1, "error out"=w124:errorcluster)  [unwired: 3 in]
                n643 = call "IMAQ AVI Create"("Compression Filter"="Microsoft Video 1", "Frames Per Second"=w107, "AVI Path"=w104) -> ("Avi Refnum"=w128:T5)  [unwired: 7 in, 1 out]
                n644 = Array Size(array=w105) -> (size(s)=w129:i32)
                n645 = for {
                  N: w129 -> [_]
                  tunnel: w128 -> [w138]
                  tunnel: w111 -> [w132]
                  tunnel: w125 -> [w140]
                  tunnel: w124 -> [w139]
                  tunnel: [w133] -> w123
                  tunnel: [FALSE ("Play")] -> w102
                  tunnel: ["Writing complete" ("message")] -> w122
                  tunnel: [w131] -> w121
                  tunnel: [w135] -> w120
                  tunnel: w105 -> [w134] mode=indexing
                  i -> [w130]
                  n646 = call "IMAQ AVI Read Frame"("error in (no error)"=w139, "Frame Number"=w134, "Image"=w140, "Avi Refnum"=w132) -> ("error out"=w141:errorcluster, "Image Out"=w135:T1, "Avi Refnum (duplicate)"=w131:T5)  [unwired: 4 in, 1 out]
                  n647 = call "IMAQ AVI Write Frame"("error in (no error)"=w141, "Image"=w135, "Avi Refnum"=w138) -> ("Avi Refnum (duplicate)"=w133:T5)  [unwired: 7 in, 1 out]
                  "writing" <- w130
                }
                n648 = call "IMAQ AVI Close"("Avi Refnum"=w123) -> ()  [unwired: 10 in, 1 out]
                n649 = call "IMAQ AVI Close"("Avi Refnum"=w121) -> ("error out"=w119:errorcluster)  [unwired: 10 in]
                n650 = property on="writing" class="Slide (strict)"("Visible"=w102) -> ()  [unwired: 2 in, 2 out]
                n651 = local write "write file"(w102) -> ()
                n652 = One Button Dialog(message=w122) -> ()  [unwired: 1 in, 1 out]
                n653 = call "IMAQ Dispose"("Image"=w120, "error in (no error)"=w119) -> ()  [unwired: 4 in, 1 out]
              }
            }
          }
        }
        n654 = case shown="True" "REPORT" {
          frame False {
          }
          frame True {
            w157 = TRUE ("open new instance (false)")
            n655 = Automation Open(Automation Refnum="Word._Application", 9:w157) -> (Automation Refnum=w148:refnum<k7>, error out=w149:errorcluster)  [unwired: 2 in]
            n656 = property class="_Application"(reference=w148, error in=w149, "Visible"=w157) -> (reference out=w150:refnum<k7>, error out=w151:errorcluster)
            n657 = Current VI's Path() -> (path=w155:path)
            n658 = local write "REPORT"(FALSE ("REPORT")) -> ()
            n659 = Strip Path(path=w155) -> (stripped path=w156:path)  [unwired: 1 out]
            n660 = One Button Dialog(message="Right-click on the white strip on the LEFT of the data area to copy the data") -> ()  [unwired: 1 in, 1 out]
            n661 = Build Path(base path=w156, name or relative path="BStAT report.doc") -> (appended path=w142:path)
            n662 = property class="_Application"(reference=w150, error in=w151) -> (error out=w153:errorcluster, "Documents"=w152:refnum<k7>)  [unwired: 1 out]
            n663 = invoke class="Documents" method="Open"(reference=w152, error in=w153, "FileName"=w142, "ReadOnly"=TRUE, "Visible"=TRUE) -> ()  [unwired: 14 in, 19 out]
          }
        }
      }
      frame True {
        w1044 = u32 0 ("S_frame")
        n664 = local write "Drag control"(w1044) -> ()
        n665 = local write "START"(FALSE ("START")) -> ()
        n666 = stacked-sequence {
          frame #0 {
            w1052 = 0 ("p2code")
            w1060 = T4 4 items=["Grayscale (U8)", "Grayscale (I16)", "Grayscale (SGL)", "Complex (CSG)", "RGB (U32)", "HSL (U32)", "RGB (U64)"] ("Image Type")
            n667 = local read "Video file"() -> (w1046:path)
            n668 = call "IMAQ Create"("Image Name"="setup", "Image Type"=w1060) -> ("New Image"=w1058:T1, "error out"=w1056:errorcluster)  [unwired: 3 in]
            n669 = call "IMAQ AVI Open"("AVI Path"=w1046) -> ("Avi Refnum"=w1061:T5)  [unwired: 9 in, 1 out]
            n670 = call "IMAQ AVI Get Info"("Avi Refnum"=w1061) -> ("Number of Frames"=w1062:u32, "Avi Refnum (duplicate)"=w1054:T5, "Frame Data"=w1047:T6)  [unwired: 6 in, 2 out]
            n671 = while {
              tunnel: w1054 -> [w1072]
              tunnel: w1058 -> [w1071]
              tunnel: w1056 -> [w1070]
              tunnel: [FALSE ("Visible")] -> w1049
              tunnel: [w1067] -> w1057
              tunnel: [w1066] -> w1053
              stop <- "Start Coding" stop-if-true
              w1065 = TRUE ("Visible")
              n672 = while {
                tunnel: "Drag control" -> [w1078]
                stop <- w1076 stop-if-true
                n673 = local read "Drag control"() -> (w1073:u32)
                n674 = Not Equal?(x=w1078, y=w1073) -> (x != y?=w1075:bool)
                n675 = case shown="False" "F_Fr" {
                  tunnel: w1078 -> [_ w1081]
                  frame False {
                  }
                  frame True {
                    n676 = local write "F_frame"(w1081) -> ()
                    n677 = local write "F_Fr"(FALSE ("F_Fr")) -> ()
                  }
                }
                n678 = case shown="False" "S_Fr" {
                  tunnel: w1078 -> [_ w1083]
                  frame False {
                  }
                  frame True {
                    n679 = local write "S_frame"(w1083) -> ()
                    n680 = local write "S_Fr"(FALSE ("S_Fr")) -> ()
                  }
                }
                n681 = local read "Start Coding"() -> (w1074:bool)
                n682 = Or(x=w1075, y=w1074) -> (x .or. y?=w1076:bool)
              }
              n683 = call "IMAQ AVI Read Frame"("error in (no error)"=w1070, "Frame Number"="Drag control", "Image"=w1071, "Avi Refnum"=w1072) -> ("Image Out"=→"Video":T1, "Avi Refnum (duplicate)"=w1067:T5)  [unwired: 4 in, 2 out]
              n684 = property on="Drag control" class="Slide (strict)"("Visible"=w1065) -> ()  [unwired: 2 in, 2 out]
              n685 = property on="S_frame" class="DigNum (strict)"("Visible"=w1065) -> ()  [unwired: 2 in, 2 out]
              n686 = property on="Start Coding" class="Bool (strict)"("Visible"=w1065) -> ()  [unwired: 2 in, 2 out]
              n687 = property on="S_Fr" class="Bool (strict)"("Visible"=w1065) -> ()  [unwired: 2 in, 2 out]
              n688 = property on="F_frame" class="DigNum (strict)"("Visible"=w1065) -> ()  [unwired: 2 in, 2 out]
              n689 = property on="F_Fr" class="Bool (strict)"("Visible"=w1065) -> ()  [unwired: 2 in, 2 out]
              n690 = local read "S_frame"() -> (w1066:u32)
            }
            n691 = Decrement(x=w1062) -> (x-1=w1051:u32)
            n692 = property on="Drag control" class="Slide (strict)"("Scale.Maximum"=w1051, "Scale.Minimum"=0.0 ("Scale.Range:Minimum")) -> ()  [unwired: 2 in, 2 out]
            n693 = Unbundle By Name(w1047) -> ("framesPerSecond"=→"framesPerSecond":u32)
            n694 = One Button Dialog(message="Please Select the start and end points\nof the video for coding ") -> ()  [unwired: 1 in, 1 out]
            n695 = call "IMAQ AVI Close"("Avi Refnum"=w1057) -> ()  [unwired: 10 in, 1 out]
            n696 = local write "Start Coding"(w1049) -> ()
            n697 = local write "p2code"(w1052) -> ()
            n698 = local write "p1code"(w1052) -> ()
            n699 = property on="S_frame" class="DigNum (strict)"("Visible"=w1049) -> ()  [unwired: 2 in, 2 out]
            n700 = property on="Start Coding" class="Bool (strict)"("Visible"=w1049) -> ()  [unwired: 2 in, 2 out]
            n701 = property on="S_Fr" class="Bool (strict)"("Visible"=w1049) -> ()  [unwired: 2 in, 2 out]
            n702 = property on="F_frame" class="DigNum (strict)"("Visible"=w1049) -> ()  [unwired: 2 in, 2 out]
            n703 = property on="F_Fr" class="Bool (strict)"("Visible"=w1049) -> ()  [unwired: 2 in, 2 out]
            n704 = local write "Progress..."(w1053) -> ()
          }
          frame #1 {
            w1101 = "\r"
            w1097 = TRUE ("Visible")
            w1095 = TRUE ("Visible")
            w1114 = T4 4 items=["Grayscale (U8)", "Grayscale (I16)", "Grayscale (SGL)", "Complex (CSG)", "RGB (U32)", "HSL (U32)", "RGB (U64)"] ("Image Type")
            n705 = local read "Video file"() -> (w1103:path)
            n706 = call "IMAQ Create"("Image Name"="code", "Image Type"=w1114) -> ("New Image"=w1113:T1, "error out"=w1112:errorcluster)  [unwired: 3 in]
            n707 = call "IMAQ AVI Open"("AVI Path"=w1103) -> ("Avi Refnum"=w1111:T5)  [unwired: 9 in, 1 out]
            n708 = while {
              tunnel: w1113 -> [w1146]
              tunnel: w1112 -> [w1145]
              tunnel: w1111 -> [w1151]
              tunnel: [FALSE] -> w1098
              tunnel: [w1153] -> w1086
              tunnel: [w1150] -> w1099
              tunnel: [w1129] -> w1087
              tunnel: [w1127] -> w1085
              stop <- w1126 stop-if-true
              n709 = case shown="True" "switch sides" {
                frame False {
                }
                frame True {
                  n710 = stacked-sequence {
                    frame #0 {
                      n711 = property on="Name 1" class="Str"() -> ("Position"=w1200:T7)  [unwired: 2 in, 2 out]
                      n712 = property on="Name 2" class="Str"() -> ("Position"=w1199:T7)  [unwired: 2 in, 2 out]
                      n713 = property on="Name 3" class="Str"() -> ("Position"=w1198:T7)  [unwired: 2 in, 2 out]
                      n714 = property on="Name 4" class="Str"() -> ("Position"=w1197:T7)  [unwired: 2 in, 2 out]
                      n715 = property on="Player 1" class="Bool (strict)"() -> ("Position"=w1195:T7)  [unwired: 2 in, 2 out]
                      n716 = property on="Player 2" class="Bool (strict)"() -> ("Position"=w1196:T7)  [unwired: 2 in, 2 out]
                      n717 = property on="Player 3" class="Bool (strict)"() -> ("Position"=w1194:T7)  [unwired: 2 in, 2 out]
                      n718 = property on="Player 4" class="Bool (strict)"() -> ("Position"=w1193:T7)  [unwired: 2 in, 2 out]
                      n719 = property on="Score1" class="DigNum (strict)"() -> ("Position"=w1192:T7)  [unwired: 2 in, 2 out]
                      n720 = property on="Score2" class="DigNum (strict)"() -> ("Position"=w1191:T7)  [unwired: 2 in, 2 out]
                      n721 = property on="E1" class="Bool (strict)"() -> ("Position"=w1190:T7)  [unwired: 2 in, 2 out]
                      n722 = property on="E2" class="Bool (strict)"() -> ("Position"=w1189:T7)  [unwired: 2 in, 2 out]
                      n723 = property on="W1" class="Bool (strict)"() -> ("Position"=w1185:T7)  [unwired: 2 in, 2 out]
                      n724 = property on="W2" class="Bool (strict)"() -> ("Position"=w1186:T7)  [unwired: 2 in, 2 out]
                      n725 = property on="Pause 1" class="Bool (strict)"() -> ("Position"=w1187:T7)  [unwired: 2 in, 2 out]
                      n726 = property on="Pause 2" class="Bool (strict)"() -> ("Position"=w1188:T7)  [unwired: 2 in, 2 out]
                      n727 = Bundle("Position"=w1200, "Position"=w1199, "Position"=w1198, "Position"=w1197, "Position"=w1195, "Position"=w1196, "Position"=w1194, "Position"=w1193) -> (w1184:T8)  [unwired: 1 in]
                      n728 = Bundle("Position"=w1192, "Position"=w1191, "Position"=w1190, "Position"=w1189, "Position"=w1185, "Position"=w1186, "Position"=w1187, "Position"=w1188) -> (w1183:T8)  [unwired: 1 in]
                      n729 = Unbundle(w1183) -> ("Position"=w1182:T7, "Position"=w1181:T7, "Position"=w1180:T7, "Position"=w1179:T7, "Position"=w1178:T7, "Position"=w1177:T7, "Position"=w1176:T7, "Position"=w1175:T7)
                      n730 = Unbundle(w1184) -> ("Position"=w1174:T7, "Position"=w1173:T7, "Position"=w1172:T7, "Position"=w1171:T7, "Position"=w1170:T7, "Position"=w1169:T7, "Position"=w1168:T7, "Position"=w1167:T7)
                      n731 = property on="Score2" class="DigNum (strict)"("Position"=w1182) -> ()  [unwired: 2 in, 2 out]
                      n732 = property on="Score1" class="DigNum (strict)"("Position"=w1181) -> ()  [unwired: 2 in, 2 out]
                      n733 = property on="E2" class="Bool (strict)"("Position"=w1180) -> ()  [unwired: 2 in, 2 out]
                      n734 = property on="E1" class="Bool (strict)"("Position"=w1179) -> ()  [unwired: 2 in, 2 out]
                      n735 = property on="W2" class="Bool (strict)"("Position"=w1178) -> ()  [unwired: 2 in, 2 out]
                      n736 = property on="W1" class="Bool (strict)"("Position"=w1177) -> ()  [unwired: 2 in, 2 out]
                      n737 = property on="Pause 2" class="Bool (strict)"("Position"=w1176) -> ()  [unwired: 2 in, 2 out]
                      n738 = property on="Pause 1" class="Bool (strict)"("Position"=w1175) -> ()  [unwired: 2 in, 2 out]
                      n739 = property on="Name 3" class="Str"("Position"=w1174) -> ()  [unwired: 2 in, 2 out]
                      n740 = property on="Name 4" class="Str"("Position"=w1173) -> ()  [unwired: 2 in, 2 out]
                      n741 = property on="Name 1" class="Str"("Position"=w1172) -> ()  [unwired: 2 in, 2 out]
                      n742 = property on="Name 2" class="Str"("Position"=w1171) -> ()  [unwired: 2 in, 2 out]
                      n743 = property on="Player 3" class="Bool (strict)"("Position"=w1170) -> ()  [unwired: 2 in, 2 out]
                      n744 = property on="Player 4" class="Bool (strict)"("Position"=w1169) -> ()  [unwired: 2 in, 2 out]
                      n745 = property on="Player 1" class="Bool (strict)"("Position"=w1168) -> ()  [unwired: 2 in, 2 out]
                      n746 = property on="Player 2" class="Bool (strict)"("Position"=w1167) -> ()  [unwired: 2 in, 2 out]
                    }
                    frame #1 {
                      n747 = property on="TL 3" class="Bool (strict)"() -> ("Position"=w1226:T7)  [unwired: 2 in, 2 out]
                      n748 = property on="TL 2" class="Bool (strict)"() -> ("Position"=w1225:T7)  [unwired: 2 in, 2 out]
                      n749 = property on="ML 3" class="Bool (strict)"() -> ("Position"=w1224:T7)  [unwired: 2 in, 2 out]
                      n750 = property on="ML 2" class="Bool (strict)"() -> ("Position"=w1223:T7)  [unwired: 2 in, 2 out]
                      n751 = property on="BL 3" class="Bool (strict)"() -> ("Position"=w1222:T7)  [unwired: 2 in, 2 out]
                      n752 = property on="BL 2" class="Bool (strict)"() -> ("Position"=w1221:T7)  [unwired: 2 in, 2 out]
                      n753 = Bundle("Position"=w1226, "Position"=w1225, "Position"=w1224, "Position"=w1223, "Position"=w1222, "Position"=w1221) -> (w1214:T9)  [unwired: 1 in]
                      n754 = property on="TCL 3" class="Bool (strict)"() -> ("Position"=w1220:T7)  [unwired: 2 in, 2 out]
                      n755 = property on="TCL 2" class="Bool (strict)"() -> ("Position"=w1219:T7)  [unwired: 2 in, 2 out]
                      n756 = property on="MCL 3" class="Bool (strict)"() -> ("Position"=w1218:T7)  [unwired: 2 in, 2 out]
                      n757 = property on="MCL 2" class="Bool (strict)"() -> ("Position"=w1217:T7)  [unwired: 2 in, 2 out]
                      n758 = property on="BCL 3" class="Bool (strict)"() -> ("Position"=w1216:T7)  [unwired: 2 in, 2 out]
                      n759 = property on="BCL 2" class="Bool (strict)"() -> ("Position"=w1215:T7)  [unwired: 2 in, 2 out]
                      n760 = Bundle("Position"=w1220, "Position"=w1219, "Position"=w1218, "Position"=w1217, "Position"=w1216, "Position"=w1215) -> (w1213:T9)  [unwired: 1 in]
                      n761 = Unbundle(w1213) -> ("Position"=w1207:T7, "Position"=w1208:T7, "Position"=w1209:T7, "Position"=w1210:T7, "Position"=w1211:T7, "Position"=w1212:T7)
                      n762 = Unbundle(w1214) -> ("Position"=w1206:T7, "Position"=w1205:T7, "Position"=w1204:T7, "Position"=w1203:T7, "Position"=w1202:T7, "Position"=w1201:T7)
                      n763 = property on="TCL 2" class="Bool (strict)"("Position"=w1207) -> ()  [unwired: 2 in, 2 out]
                      n764 = property on="TCL 3" class="Bool (strict)"("Position"=w1208) -> ()  [unwired: 2 in, 2 out]
                      n765 = property on="MCL 2" class="Bool (strict)"("Position"=w1209) -> ()  [unwired: 2 in, 2 out]
                      n766 = property on="MCL 3" class="Bool (strict)"("Position"=w1210) -> ()  [unwired: 2 in, 2 out]
                      n767 = property on="BCL 2" class="Bool (strict)"("Position"=w1211) -> ()  [unwired: 2 in, 2 out]
                      n768 = property on="BCL 3" class="Bool (strict)"("Position"=w1212) -> ()  [unwired: 2 in, 2 out]
                      n769 = property on="TL 2" class="Bool (strict)"("Position"=w1206) -> ()  [unwired: 2 in, 2 out]
                      n770 = property on="TL 3" class="Bool (strict)"("Position"=w1205) -> ()  [unwired: 2 in, 2 out]
                      n771 = property on="ML 2" class="Bool (strict)"("Position"=w1204) -> ()  [unwired: 2 in, 2 out]
                      n772 = property on="ML 3" class="Bool (strict)"("Position"=w1203) -> ()  [unwired: 2 in, 2 out]
                      n773 = property on="BL 2" class="Bool (strict)"("Position"=w1202) -> ()  [unwired: 2 in, 2 out]
                      n774 = property on="BL 3" class="Bool (strict)"("Position"=w1201) -> ()  [unwired: 2 in, 2 out]
                    }
                    frame #2 {
                      n775 = property on="TC 3" class="Bool (strict)"() -> ("Position"=w1252:T7)  [unwired: 2 in, 2 out]
                      n776 = property on="TC 2" class="Bool (strict)"() -> ("Position"=w1251:T7)  [unwired: 2 in, 2 out]
                      n777 = property on="MC 3" class="Bool (strict)"() -> ("Position"=w1250:T7)  [unwired: 2 in, 2 out]
                      n778 = property on="MC 2" class="Bool (strict)"() -> ("Position"=w1249:T7)  [unwired: 2 in, 2 out]
                      n779 = property on="BC 3" class="Bool (strict)"() -> ("Position"=w1248:T7)  [unwired: 2 in, 2 out]
                      n780 = property on="BC 2" class="Bool (strict)"() -> ("Position"=w1247:T7)  [unwired: 2 in, 2 out]
                      n781 = property on="TCR 3" class="Bool (strict)"() -> ("Position"=w1246:T7)  [unwired: 2 in, 2 out]
                      n782 = property on="TCR 2" class="Bool (strict)"() -> ("Position"=w1245:T7)  [unwired: 2 in, 2 out]
                      n783 = property on="MCR  3" class="Bool (strict)"() -> ("Position"=w1244:T7)  [unwired: 2 in, 2 out]
                      n784 = property on="MCR 2" class="Bool (strict)"() -> ("Position"=w1243:T7)  [unwired: 2 in, 2 out]
                      n785 = property on="BCR 3" class="Bool (strict)"() -> ("Position"=w1242:T7)  [unwired: 2 in, 2 out]
                      n786 = property on="BCR 2" class="Bool (strict)"() -> ("Position"=w1241:T7)  [unwired: 2 in, 2 out]
                      n787 = Bundle("Position"=w1252, "Position"=w1251, "Position"=w1250, "Position"=w1249, "Position"=w1248, "Position"=w1247) -> (w1240:T9)  [unwired: 1 in]
                      n788 = Bundle("Position"=w1246, "Position"=w1245, "Position"=w1244, "Position"=w1243, "Position"=w1242, "Position"=w1241) -> (w1239:T9)  [unwired: 1 in]
                      n789 = Unbundle(w1239) -> ("Position"=w1238:T7, "Position"=w1237:T7, "Position"=w1236:T7, "Position"=w1235:T7, "Position"=w1234:T7, "Position"=w1233:T7)
                      n790 = Unbundle(w1240) -> ("Position"=w1227:T7, "Position"=w1228:T7, "Position"=w1229:T7, "Position"=w1230:T7, "Position"=w1231:T7, "Position"=w1232:T7)
                      n791 = property on="TCR 2" class="Bool (strict)"("Position"=w1238) -> ()  [unwired: 2 in, 2 out]
                      n792 = property on="TCR 3" class="Bool (strict)"("Position"=w1237) -> ()  [unwired: 2 in, 2 out]
                      n793 = property on="MCR 2" class="Bool (strict)"("Position"=w1236) -> ()  [unwired: 2 in, 2 out]
                      n794 = property on="MCR  3" class="Bool (strict)"("Position"=w1235) -> ()  [unwired: 2 in, 2 out]
                      n795 = property on="BCR 2" class="Bool (strict)"("Position"=w1234) -> ()  [unwired: 2 in, 2 out]
                      n796 = property on="BCR 3" class="Bool (strict)"("Position"=w1233) -> ()  [unwired: 2 in, 2 out]
                      n797 = property on="TC 2" class="Bool (strict)"("Position"=w1227) -> ()  [unwired: 2 in, 2 out]
                      n798 = property on="TC 3" class="Bool (strict)"("Position"=w1228) -> ()  [unwired: 2 in, 2 out]
                      n799 = property on="MC 2" class="Bool (strict)"("Position"=w1229) -> ()  [unwired: 2 in, 2 out]
                      n800 = property on="MC 3" class="Bool (strict)"("Position"=w1230) -> ()  [unwired: 2 in, 2 out]
                      n801 = property on="BC 2" class="Bool (strict)"("Position"=w1231) -> ()  [unwired: 2 in, 2 out]
                      n802 = property on="BC 3" class="Bool (strict)"("Position"=w1232) -> ()  [unwired: 2 in, 2 out]
                    }
                    frame #3 {
                      n803 = property on="TR 3" class="Bool (strict)"() -> ("Position"=w1275:T7)  [unwired: 2 in, 2 out]
                      n804 = property on="TR 2" class="Bool (strict)"() -> ("Position"=w1274:T7)  [unwired: 2 in, 2 out]
                      n805 = property on="MR  3" class="Bool (strict)"() -> ("Position"=w1273:T7)  [unwired: 2 in, 2 out]
                      n806 = property on="MR  2" class="Bool (strict)"() -> ("Position"=w1272:T7)  [unwired: 2 in, 2 out]
                      n807 = property on="BR 3" class="Bool (strict)"() -> ("Position"=w1271:T7)  [unwired: 2 in, 2 out]
                      n808 = property on="BR 2" class="Bool (strict)"() -> ("Position"=w1270:T7)  [unwired: 2 in, 2 out]
                      n809 = property on="S1" class="Bool (strict)"() -> ("Position"=w1262:T7)  [unwired: 2 in, 2 out]
                      n810 = property on="S2" class="Bool (strict)"() -> ("Position"=w1261:T7)  [unwired: 2 in, 2 out]
                      n811 = property on="S3" class="Bool (strict)"() -> ("Position"=w1260:T7)  [unwired: 2 in, 2 out]
                      n812 = property on="S4" class="Bool (strict)"() -> ("Position"=w1259:T7)  [unwired: 2 in, 2 out]
                      n813 = Bundle("Position"=w1275, "Position"=w1274, "Position"=w1273, "Position"=w1272, "Position"=w1271, "Position"=w1270) -> (w1269:T9)  [unwired: 1 in]
                      n814 = Bundle("Position"=w1262, "Position"=w1261, "Position"=w1260, "Position"=w1259) -> (w1258:T10)  [unwired: 1 in]
                      n815 = Unbundle(w1269) -> ("Position"=w1263:T7, "Position"=w1264:T7, "Position"=w1268:T7, "Position"=w1267:T7, "Position"=w1266:T7, "Position"=w1265:T7)
                      n816 = Unbundle(w1258) -> ("Position"=w1257:T7, "Position"=w1256:T7, "Position"=w1255:T7, "Position"=w1254:T7)
                      n817 = property on="TR 2" class="Bool (strict)"("Position"=w1263) -> ()  [unwired: 2 in, 2 out]
                      n818 = property on="TR 3" class="Bool (strict)"("Position"=w1264) -> ()  [unwired: 2 in, 2 out]
                      n819 = property on="MR  2" class="Bool (strict)"("Position"=w1268) -> ()  [unwired: 2 in, 2 out]
                      n820 = property on="MR  3" class="Bool (strict)"("Position"=w1267) -> ()  [unwired: 2 in, 2 out]
                      n821 = property on="BR 2" class="Bool (strict)"("Position"=w1266) -> ()  [unwired: 2 in, 2 out]
                      n822 = property on="BR 3" class="Bool (strict)"("Position"=w1265) -> ()  [unwired: 2 in, 2 out]
                      n823 = local write "switch sides"(FALSE ("court")) -> ()
                      n824 = property on="S3" class="Bool (strict)"("Position"=w1257) -> ()  [unwired: 2 in, 2 out]
                      n825 = property on="S4" class="Bool (strict)"("Position"=w1256) -> ()  [unwired: 2 in, 2 out]
                      n826 = property on="S1" class="Bool (strict)"("Position"=w1255) -> ()  [unwired: 2 in, 2 out]
                      n827 = property on="S2" class="Bool (strict)"("Position"=w1254) -> ()  [unwired: 2 in, 2 out]
                    }
                  }
                }
              }
              n828 = Increment(x="Progress...") -> (x+1=w1152:i32)
              n829 = call "IMAQ AVI Read Frame"("error in (no error)"=w1145, "Frame Number"=w1152, "Image"=w1146, "Avi Refnum"=w1151) -> ("Image Out"=w1143:T1)  [unwired: 4 in, 3 out]
              n830 = local write "Video"(w1143) -> ()
              n831 = Add(x=9, y=w1152) -> (x+y=w1155:i32)
              n832 = local read "F_frame"() -> (w1156:u32)
              n833 = local read "framesPerSecond"() -> (w1138:u32)
              n834 = Less Or Equal?(x=w1156, y=w1155) -> (x <= y?=w1142:bool)
              n835 = Select(t=w1155, s="fast forward", f=w1152) -> (s? t:f=w1140:i32)
              n836 = Select(t="Progress...", s=w1142, f=w1140) -> (s? t:f=w1141:i32)
              n837 = Divide(x=1000.0, y="playback speed") -> (x/y=w1159:dbl)
              n838 = local write "Progress..."(w1141) -> ()
              n839 = Divide(x=w1159, y=w1138) -> (x/y=w1137:dbl)
              n840 = Wait (ms)(milliseconds to wait=w1137) -> ()  [unwired: 1 out]
              n841 = Compound Arithmetic op=OR("Pause 1", "Pause 2", "Pause 3") -> (w1154:bool)
              n842 = case shown="True" w1154 {
                tunnel: w1152 -> [w1288 w1413]
                tunnel: [w1287 w1399] -> w1153
                tunnel: w1152 -> [_ w1416]
                tunnel: w1151 -> [w1285 w1415]
                tunnel: [w1285 w1412] -> w1150
                tunnel: "Pause 1" -> [_ w1411]
                tunnel: "Pause 2" -> [_ w1352]
                tunnel: w1137 -> [_ w1407]
                frame False {
                  n843 = local read "W1"() -> (w1284:bool)
                  n844 = local read "W2"() -> (w1282:bool)
                  n845 = local read "E1"() -> (w1283:bool)
                  n846 = local read "E2"() -> (w1281:bool)
                  n847 = Or(x=w1284, y=w1283) -> (x .or. y?=w1280:bool)
                  n848 = Or(x=w1282, y=w1281) -> (x .or. y?=w1279:bool)
                  n849 = Boolean To (0,1)(Boolean=w1280) -> (0, 1=w1277:i16)
                  n850 = Select(t=2.0, s=w1279, f=w1277) -> (s? t:f=w1276:dbl)
                  n851 = case shown="0, Default" w1276 {
                    tunnel: w1288 -> [_ _ _]
                    tunnel: [w1291 w1320 w1323] -> w1287
                    tunnel: [FALSE FALSE FALSE] -> w1286
                    frame 0, Default {
                      w1289 = FALSE ("4 6")
                      n852 = local write "1 6"(w1289) -> ()
                      n853 = local write "2 6"(w1289) -> ()
                      n854 = local write "3 6"(w1289) -> ()
                      n855 = local write "4 6"(w1289) -> ()
                      n856 = local write "5 6"(w1289) -> ()
                      n857 = local write "6 6"(w1289) -> ()
                      n858 = local write "7 6"(w1289) -> ()
                      n859 = local write "8 6"(w1289) -> ()
                      n860 = local write "9 6"(w1289) -> ()
                      n861 = local write "10 6"(w1289) -> ()
                      n862 = local write "1 5"(w1289) -> ()
                      n863 = local write "2 5"(w1289) -> ()
                      n864 = local write "3 5"(w1289) -> ()
                      n865 = local write "4 5"(w1289) -> ()
                      n866 = local write "5 5"(w1289) -> ()
                      n867 = local write "6 5"(w1289) -> ()
                      n868 = local write "7 5"(w1289) -> ()
                      n869 = local write "8 5"(w1289) -> ()
                      n870 = local write "9 5"(w1289) -> ()
                      n871 = local write "10 5"(w1289) -> ()
                      n872 = local write "1 4"(w1289) -> ()
                      n873 = local write "2 4"(w1289) -> ()
                      n874 = local write "3 4"(w1289) -> ()
                      n875 = local write "4 4"(w1289) -> ()
                      n876 = local write "5 4"(w1289) -> ()
                      n877 = local write "6 4"(w1289) -> ()
                      n878 = local write "7 4"(w1289) -> ()
                      n879 = local write "8 4"(w1289) -> ()
                      n880 = local write "9 4"(w1289) -> ()
                      n881 = local write "10 4"(w1289) -> ()
                      n882 = local write "1 3"(w1289) -> ()
                      n883 = local write "2 3"(w1289) -> ()
                      n884 = local write "3 3"(w1289) -> ()
                      n885 = local write "4 3"(w1289) -> ()
                      n886 = local write "5 3"(w1289) -> ()
                      n887 = local write "6 3"(w1289) -> ()
                      n888 = local write "7 3"(w1289) -> ()
                      n889 = local write "8 3"(w1289) -> ()
                      n890 = local write "9 3"(w1289) -> ()
                      n891 = local write "10 3"(w1289) -> ()
                      n892 = local write "1 2"(w1289) -> ()
                      n893 = local write "2 2"(w1289) -> ()
                      n894 = local write "3 2"(w1289) -> ()
                      n895 = local write "4 2"(w1289) -> ()
                      n896 = local write "5 2"(w1289) -> ()
                      n897 = local write "6 2"(w1289) -> ()
                      n898 = local write "7 2"(w1289) -> ()
                      n899 = local write "8 2"(w1289) -> ()
                      n900 = local write "9 2"(w1289) -> ()
                      n901 = local write "10 2"(w1289) -> ()
                      n902 = local write "1"(w1289) -> ()
                      n903 = local write "2"(w1289) -> ()
                      n904 = local write "3"(w1289) -> ()
                      n905 = local write "4"(w1289) -> ()
                      n906 = local write "5"(w1289) -> ()
                      n907 = local write "6"(w1289) -> ()
                      n908 = local write "7"(w1289) -> ()
                      n909 = local write "8"(w1289) -> ()
                      n910 = local write "9"(w1289) -> ()
                      n911 = local write "10"(w1289) -> ()
                      n912 = local write "BCL 3"(w1289) -> ()
                      n913 = local write "BCL 2"(w1289) -> ()
                      n914 = local write "BL 3"(w1289) -> ()
                      n915 = local write "BL 2"(w1289) -> ()
                      n916 = local write "BC 3"(w1289) -> ()
                      n917 = local write "BC 2"(w1289) -> ()
                      n918 = local write "BCR 3"(w1289) -> ()
                      n919 = local write "BCR 2"(w1289) -> ()
                      n920 = local write "Player 1"(w1289) -> ()
                      n921 = local write "Player 2"(w1289) -> ()
                      n922 = local write "Player 3"(w1289) -> ()
                      n923 = local write "Player 4"(w1289) -> ()
                      n924 = local write "BR 2"(w1289) -> ()
                      n925 = local write "BR 3"(w1289) -> ()
                      n926 = local write "W1"(w1289) -> ()
                      n927 = local write "W2"(w1289) -> ()
                      n928 = local write "E1"(w1289) -> ()
                      n929 = local write "E2"(w1289) -> ()
                      n930 = local write "TCL 3"(w1289) -> ()
                      n931 = local write "TCL 2"(w1289) -> ()
                      n932 = local write "TL 3"(w1289) -> ()
                      n933 = local write "TL 2"(w1289) -> ()
                      n934 = local write "TC 2"(w1289) -> ()
                      n935 = local write "TC 3"(w1289) -> ()
                      n936 = local write "TCR 3"(w1289) -> ()
                      n937 = local write "TCR 2"(w1289) -> ()
                      n938 = local write "TR 2"(w1289) -> ()
                      n939 = local write "TR 3"(w1289) -> ()
                      n940 = local write "MCL 3"(w1289) -> ()
                      n941 = local write "MCL 2"(w1289) -> ()
                      n942 = local write "ML 3"(w1289) -> ()
                      n943 = local write "ML 2"(w1289) -> ()
                      n944 = local write "MC 2"(w1289) -> ()
                      n945 = local write "MC 3"(w1289) -> ()
                      n946 = local write "MR  2"(w1289) -> ()
                      n947 = local write "MR  3"(w1289) -> ()
                      n948 = local write "MCR  3"(w1289) -> ()
                      n949 = local write "MCR 2"(w1289) -> ()
                      n950 = local write "S1"(w1289) -> ()
                      n951 = local write "S2"(w1289) -> ()
                      n952 = local write "S3"(w1289) -> ()
                      n953 = local write "S4"(w1289) -> ()
                      n954 = local write "1"(w1289) -> ()
                      n955 = local write "2"(w1289) -> ()
                      n956 = local write "3"(w1289) -> ()
                      n957 = local write "4"(w1289) -> ()
                      n958 = local write "5"(w1289) -> ()
                      n959 = local read "coding"() -> (w1291:i32[][])
                    }
                    frame 1 {
                      n960 = local read "W1"() -> (w1314:bool)
                      n961 = local read "W2"() -> (w1315:bool)
                      n962 = local read "E1"() -> (w1316:bool)
                      n963 = local read "E2"() -> (w1317:bool)
                      n964 = Boolean To (0,1)(Boolean=w1314) -> (0, 1=w1306:i16)
                      n965 = Boolean To (0,1)(Boolean=w1315) -> (0, 1=w1305:i16)
                      n966 = Boolean To (0,1)(Boolean=w1316) -> (0, 1=w1300:i16)
                      n967 = Boolean To (0,1)(Boolean=w1317) -> (0, 1=w1299:i16)
                      n968 = Or(x=w1314, y=w1317) -> (x .or. y?=w1313:bool)
                      n969 = Or(x=w1315, y=w1316) -> (x .or. y?=w1312:bool)
                      n970 = local read "Score2"() -> (w1292:i32)
                      n971 = local read "Score1"() -> (w1318:i32)
                      n972 = Increment(x=w1318) -> (x+1=w1311:i32)
                      n973 = Increment(x=w1292) -> (x+1=w1310:i32)
                      n974 = Select(t=w1310, s=w1312, f=w1292) -> (s? t:f=w1293:i32)
                      n975 = Select(t=w1311, s=w1313, f=w1318) -> (s? t:f=w1295:i32)
                      n976 = Boolean To (0,1)(Boolean=w1313) -> (0, 1=w1298:i16)
                      n977 = Boolean To (0,1)(Boolean=w1312) -> (0, 1=w1297:i16)
                      n978 = local write "Score1"(w1295) -> ()
                      n979 = local write "Score2"(w1293) -> ()
                      n980 = local read "p1code"() -> (w1308:i32)
                      n981 = local read "coding"() -> (w1319:i32[][])
                      n982 = Replace Array Subset(array=w1319, new element #1=w1306, index (row) #1=w1308, index (col) #1=31 ("disabled index (col)"), new element #2=w1305, index (row) #2=w1308, index (col) #2=32 ("disabled index (col)"), new element #3=w1300, index (row) #3=w1308, index (col) #3=33 ("disabled index (col)"), new element #4=w1299, index (row) #4=w1308, index (col) #4=34 ("disabled index (col)"), new element #5=w1298, index (row) #5=w1308, index (col) #5=35 ("disabled index (col)"), new element #6=w1297, index (row) #6=w1308, index (col) #6=36 ("disabled index (col)"), new element #7=w1295, index (row) #7=w1308, index (col) #7=37 ("disabled index (col)"), new element #8=w1293, index (row) #8=w1308, index (col) #8=38 ("disabled index (col)")) -> (w1320:i32[][])
                      n983 = local write "coding"(w1320) -> ()
                    }
                    frame 2 {
                      n984 = local read "W1"() -> (w1346:bool)
                      n985 = local read "W2"() -> (w1347:bool)
                      n986 = local read "E1"() -> (w1348:bool)
                      n987 = local read "E2"() -> (w1349:bool)
                      n988 = Boolean To (0,1)(Boolean=w1346) -> (0, 1=w1339:i16)
                      n989 = Boolean To (0,1)(Boolean=w1347) -> (0, 1=w1338:i16)
                      n990 = Boolean To (0,1)(Boolean=w1348) -> (0, 1=w1333:i16)
                      n991 = Boolean To (0,1)(Boolean=w1349) -> (0, 1=w1332:i16)
                      n992 = Or(x=w1346, y=w1349) -> (x .or. y?=w1345:bool)
                      n993 = Or(x=w1347, y=w1348) -> (x .or. y?=w1344:bool)
                      n994 = local read "Score2"() -> (w1322:i32)
                      n995 = local read "Score1"() -> (w1350:i32)
                      n996 = Increment(x=w1350) -> (x+1=w1343:i32)
                      n997 = Increment(x=w1322) -> (x+1=w1342:i32)
                      n998 = Select(t=w1342, s=w1344, f=w1322) -> (s? t:f=w1326:i32)
                      n999 = Select(t=w1343, s=w1345, f=w1350) -> (s? t:f=w1328:i32)
                      n1000 = Boolean To (0,1)(Boolean=w1345) -> (0, 1=w1331:i16)
                      n1001 = Boolean To (0,1)(Boolean=w1344) -> (0, 1=w1330:i16)
                      n1002 = local write "Score1"(w1328) -> ()
                      n1003 = local write "Score2"(w1326) -> ()
                      n1004 = local read "p2code"() -> (w1324:i32)
                      n1005 = local read "coding"() -> (w1351:i32[][])
                      n1006 = Replace Array Subset(array=w1351, new element #1=w1339, index (row) #1=w1324, index (col) #1=31 ("disabled index (col)"), new element #2=w1338, index (row) #2=w1324, index (col) #2=32 ("disabled index (col)"), new element #3=w1333, index (row) #3=w1324, index (col) #3=33 ("disabled index (col)"), new element #4=w1332, index (row) #4=w1324, index (col) #4=34 ("disabled index (col)"), new element #5=w1331, index (row) #5=w1324, index (col) #5=35 ("disabled index (col)"), new element #6=w1330, index (row) #6=w1324, index (col) #6=36 ("disabled index (col)"), new element #7=w1328, index (row) #7=w1324, index (col) #7=37 ("disabled index (col)"), new element #8=w1326, index (row) #8=w1324, index (col) #8=38 ("disabled index (col)")) -> (w1323:i32[][])
                      n1007 = local write "coding"(w1323) -> ()
                    }
                  }
                  n1008 = local write "W1"(w1286) -> ()
                  n1009 = local write "W2"(w1286) -> ()
                  n1010 = local write "E1"(w1286) -> ()
                  n1011 = local write "E2"(w1286) -> ()
                }
                frame True {
                  n1012 = stacked-sequence {
                    tunnel: [_ w1487 _ _ _ _ _ _] -> w1414
                    tunnel: w1416 -> [w1425 _ _ _ _ _ _ _]
                    tunnel: w1415 -> [w1424 _ _ _ _ _ _ _]
                    tunnel: [w1423 _ _ _ _ _ _ _] -> w1412
                    tunnel: [_ _ _ _ _ _ _ w1802] -> w1400
                    tunnel: w1411 -> [_ _ w1558 _ _ _ _ _]
                    tunnel: w1352 -> [_ _ w1557 _ _ _ _ _]
                    tunnel: w1407 -> [w1418 _ _ _ _ _ _ _]
                    tunnel: [w1417 _ _ _ _ _ _ _] -> w1398
                    tunnel: [_ w1482 _ _ _ _ _ _] -> w1397
                    tunnel: [_ w1481 _ _ _ _ _ _] -> w1396
                    tunnel: [_ w1478 _ _ _ _ _ _] -> w1395
                    tunnel: [_ w1454 _ _ _ _ _ _] -> w1394
                    tunnel: [_ w1470 _ _ _ _ _ _] -> w1393
                    tunnel: [_ w1469 _ _ _ _ _ _] -> w1392
                    tunnel: [_ w1468 _ _ _ _ _ _] -> w1391
                    tunnel: [_ w1467 _ _ _ _ _ _] -> w1390
                    tunnel: [_ w1466 _ _ _ _ _ _] -> w1389
                    tunnel: [_ w1459 _ _ _ _ _ _] -> w1388
                    tunnel: [_ w1458 _ _ _ _ _ _] -> w1387
                    tunnel: [_ w1457 _ _ _ _ _ _] -> w1386
                    tunnel: [_ w1456 _ _ _ _ _ _] -> w1385
                    tunnel: [_ w1455 _ _ _ _ _ _] -> w1384
                    tunnel: [_ _ _ w1571 _ _ _ _] -> w1383
                    tunnel: [_ _ _ w1570 _ _ _ _] -> w1382
                    tunnel: [_ _ _ w1569 _ _ _ _] -> w1381
                    tunnel: [_ _ _ _ w1651 _ _ _] -> w1380
                    tunnel: [_ _ _ _ w1650 _ _ _] -> w1379
                    tunnel: [_ _ _ _ w1649 _ _ _] -> w1378
                    tunnel: [_ _ _ _ w1648 _ _ _] -> w1377
                    tunnel: [_ _ _ _ w1647 _ _ _] -> w1376
                    tunnel: [_ _ _ _ w1646 _ _ _] -> w1375
                    tunnel: [_ _ _ _ w1645 _ _ _] -> w1374
                    tunnel: [_ _ _ _ w1644 _ _ _] -> w1373
                    tunnel: [_ _ _ _ w1643 _ _ _] -> w1372
                    tunnel: [_ _ _ _ w1642 _ _ _] -> w1371
                    tunnel: [_ _ _ _ w1641 _ _ _] -> w1370
                    tunnel: [_ _ _ _ w1640 _ _ _] -> w1369
                    tunnel: [_ _ _ _ _ _ 0 ("disabled index (col)") _] -> w1368
                    tunnel: [_ _ _ _ _ _ w1792 _] -> w1367
                    tunnel: [_ _ _ _ _ _ w1791 _] -> w1366
                    tunnel: [_ _ _ _ _ _ w1788 _] -> w1365
                    tunnel: [_ _ _ _ _ _ w1787 _] -> w1364
                    tunnel: [_ _ _ _ _ _ w1786 _] -> w1363
                    tunnel: [_ _ _ _ _ _ w1785 _] -> w1362
                    tunnel: [_ _ _ _ _ _ w1784 _] -> w1361
                    tunnel: [_ _ w1519 _ _ _ _ _] -> w1360
                    tunnel: [_ _ w1518 _ _ _ _ _] -> w1359
                    tunnel: [_ _ _ _ _ _ w1783 _] -> w1358
                    tunnel: [_ _ _ _ _ _ w1782 _] -> w1357
                    tunnel: [_ _ _ _ _ _ w1777 _] -> w1356
                    tunnel: [_ _ _ _ _ _ w1776 _] -> w1355
                    tunnel: [_ _ _ _ _ _ w1775 _] -> w1354
                    tunnel: [_ _ _ _ _ _ w1774 _] -> w1353
                    frame #0 {
                      w1421 = T4 4 items=["Grayscale (U8)", "Grayscale (I16)", "Grayscale (SGL)", "Complex (CSG)", "RGB (U32)", "HSL (U32)", "RGB (U64)"] ("Image Type")
                      n1013 = while {
                        tunnel: [FALSE] -> w1422
                        stop <- w1447 continue-if-true
                        n1014 = local read "Pause 3"() -> (w1444:bool)
                        n1015 = local read "Pause 1"() -> (w1445:bool)
                        n1016 = local read "Pause 2"() -> (w1448:bool)
                        n1017 = local read "coding"() -> (w1439:i32[][])
                        n1018 = Compound Arithmetic op=OR(w1444, w1445, w1448) -> (w1447:bool)
                        n1019 = Index Array(array=w1439, index (col)=0 ("disabled index (col)")) -> (element=w1442:i32[])  [unwired: 1 in]
                        n1020 = Array Max & Min(array=w1442) -> (max value=w1441:i32, max index (indices)=w1438:i32)  [unwired: 2 out]
                        n1021 = Wait (ms)(milliseconds to wait=10.0 ("Delay Time (s)")) -> ()  [unwired: 1 out]
                        n1022 = case shown="True" "UNDO" {
                          selector: "UNDO" -> [w1449 _]
                          tunnel: w1439 -> [_ w1453]
                          tunnel: w1438 -> [_ w1452]
                          tunnel: [w1449 FALSE] -> w1437
                          frame False {
                          }
                          frame True {
                            n1023 = Delete From Array(array=w1453, index (row)=w1452) -> (array with subset deleted=w1451:i32[][])  [unwired: 2 in, 1 out]
                            n1024 = local write "coding"(w1451) -> ()
                          }
                        }
                        n1025 = local write "Last coded"(w1441) -> ()
                        n1026 = local write "UNDO"(w1437) -> ()
                      }
                      n1027 = call "IMAQ Create"("Image Name"="code3", "Image Type"=w1421) -> ("New Image"=w1417:T1, "error out"=w1419:errorcluster)  [unwired: 3 in]
                      n1028 = for {
                        N: 25 -> [_]
                        tunnel: w1425 -> [w1434]
                        tunnel: w1424 -> [w1432]
                        tunnel: w1419 -> [w1431]
                        tunnel: w1417 -> [w1430]
                        tunnel: [w1429] -> w1423
                        tunnel: w1418 -> [w1427]
                        i -> [w1435]
                        n1029 = Add(x=w1435, y=w1434) -> (x+y=w1433:i32)
                        n1030 = call "IMAQ AVI Read Frame"("error in (no error)"=w1431, "Frame Number"=w1433, "Image"=w1430, "Avi Refnum"=w1432) -> ("Image Out"=w1428:T1, "Avi Refnum (duplicate)"=w1429:T5)  [unwired: 4 in, 2 out]
                        n1031 = local write "Video"(w1428) -> ()
                        n1032 = Wait (ms)(milliseconds to wait=w1427) -> ()  [unwired: 1 out]
                      }
                      n1033 = local write "Pause 1"(w1422) -> ()
                      n1034 = local write "Pause 2"(w1422) -> ()
                      n1035 = local write "Pause 3"(w1422) -> ()
                      n1036 = local write "UNDO"(w1422) -> ()
                    }
                    frame #1 {
                      n1037 = Or(x="ML 3", y="ML 2") -> (x .or. y?=w1493:bool)
                      n1038 = Or(x="MR  2", y="MR  3") -> (x .or. y?=w1491:bool)
                      n1039 = Or(x="MC 2", y="MC 3") -> (x .or. y?=w1492:bool)
                      n1040 = Boolean To (0,1)(Boolean=w1491) -> (0, 1=w1466:i16)
                      n1041 = Boolean To (0,1)(Boolean=w1493) -> (0, 1=w1470:i16)
                      n1042 = Boolean To (0,1)(Boolean=w1492) -> (0, 1=w1468:i16)
                      n1043 = Or(x="TCL 2", y="TCL 3") -> (x .or. y?=w1486:bool)
                      n1044 = Or(x="TCR 2", y="TCR 3") -> (x .or. y?=w1480:bool)
                      n1045 = Or(x="MCR 2", y="MCR  3") -> (x .or. y?=w1473:bool)
                      n1046 = Or(x="MCL 3", y="MCL 2") -> (x .or. y?=w1476:bool)
                      n1047 = Boolean To (0,1)(Boolean=w1480) -> (0, 1=w1478:i16)
                      n1048 = Or(x="TR 2", y="TR 3") -> (x .or. y?=w1494:bool)
                      n1049 = Boolean To (0,1)(Boolean=w1486) -> (0, 1=w1482:i16)
                      n1050 = Boolean To (0,1)(Boolean=w1473) -> (0, 1=w1467:i16)
                      n1051 = Boolean To (0,1)(Boolean=w1476) -> (0, 1=w1469:i16)
                      n1052 = Or(x="BCL 2", y="BCL 3") -> (x .or. y?=w1465:bool)
                      n1053 = Or(x="TL 3", y="TL 2") -> (x .or. y?=w1496:bool)
                      n1054 = Boolean To (0,1)(Boolean=w1494) -> (0, 1=w1454:i16)
                      n1055 = Or(x="BCR 3", y="BCR 2") -> (x .or. y?=w1462:bool)
                      n1056 = Or(x="TC 2", y="TC 3") -> (x .or. y?=w1495:bool)
                      n1057 = Boolean To (0,1)(Boolean=w1465) -> (0, 1=w1458:i16)
                      n1058 = Boolean To (0,1)(Boolean=w1496) -> (0, 1=w1487:i16)
                      n1059 = Boolean To (0,1)(Boolean=w1462) -> (0, 1=w1456:i16)
                      n1060 = Boolean To (0,1)(Boolean=w1495) -> (0, 1=w1481:i16)
                      n1061 = Or(x="BL 3", y="BL 2") -> (x .or. y?=w1490:bool)
                      n1062 = Or(x="BC 3", y="BC 2") -> (x .or. y?=w1489:bool)
                      n1063 = Or(x="BR 2", y="BR 3") -> (x .or. y?=w1488:bool)
                      n1064 = Boolean To (0,1)(Boolean=w1490) -> (0, 1=w1459:i16)
                      n1065 = Boolean To (0,1)(Boolean=w1488) -> (0, 1=w1455:i16)
                      n1066 = Boolean To (0,1)(Boolean=w1489) -> (0, 1=w1457:i16)
                    }
                    frame #2 {
                      n1067 = local read "MCR  3"() -> (w1541:bool)
                      n1068 = local read "MCL 3"() -> (w1536:bool)
                      n1069 = local read "TCR 3"() -> (w1539:bool)
                      n1070 = local read "BCR 3"() -> (w1537:bool)
                      n1071 = local read "S1"() -> (w1556:bool)
                      n1072 = local read "S2"() -> (w1555:bool)
                      n1073 = local read "MR  3"() -> (w1542:bool)
                      n1074 = local read "TCL 3"() -> (w1540:bool)
                      n1075 = local read "BCL 3"() -> (w1538:bool)
                      n1076 = local read "MC 3"() -> (w1546:bool)
                      n1077 = local read "Player 1"() -> (w1517:bool)
                      n1078 = local read "Player 2"() -> (w1516:bool)
                      n1079 = local read "ML 3"() -> (w1547:bool)
                      n1080 = local read "TC 3"() -> (w1568:bool)
                      n1081 = local read "BC 3"() -> (w1545:bool)
                      n1082 = local read "BR 3"() -> (w1544:bool)
                      n1083 = local read "TR 3"() -> (w1543:bool)
                      n1084 = local read "BL 3"() -> (w1549:bool)
                      n1085 = local read "TL 3"() -> (w1548:bool)
                      n1086 = local read "Player 4"() -> (w1514:bool)
                      n1087 = local read "Player 3"() -> (w1515:bool)
                      n1088 = Or(x=w1556, y=w1555) -> (x .or. y?=w1551:bool)
                      n1089 = Compound Arithmetic op=OR(w1549, w1548, w1547, w1568, w1546, w1545, w1544, w1543, w1542, w1541, w1540, w1539, w1538, w1537, w1536) -> (w1559:bool)
                      "P1 position" <- w1559
                      n1090 = local read "coding"() -> (w1567:i32[][])
                      n1091 = Compound Arithmetic op=OR(w1559, w1558, w1517, w1516) -> (w1553:bool)
                      n1092 = local read "MCR 2"() -> (w1530:bool)
                      n1093 = local read "MCL 2"() -> (w1535:bool)
                      n1094 = local read "TCR 2"() -> (w1532:bool)
                      n1095 = local read "BCR 2"() -> (w1534:bool)
                      n1096 = local read "MR  2"() -> (w1529:bool)
                      n1097 = local read "TCL 2"() -> (w1531:bool)
                      n1098 = local read "BCL 2"() -> (w1533:bool)
                      n1099 = local read "MC 2"() -> (w1525:bool)
                      n1100 = local read "ML 2"() -> (w1524:bool)
                      n1101 = local read "TC 2"() -> (w1521:bool)
                      n1102 = local read "BC 2"() -> (w1526:bool)
                      n1103 = local read "BR 2"() -> (w1527:bool)
                      n1104 = local read "TR 2"() -> (w1528:bool)
                      n1105 = local read "BL 2"() -> (w1522:bool)
                      n1106 = local read "TL 2"() -> (w1523:bool)
                      n1107 = Or(x=w1553, y=w1551) -> (x .or. y?=w1554:bool)
                      n1108 = Array Size(array=w1567) -> (size(s)=w1566:i32[])
                      n1109 = local read "p1code"() -> (w1563:i32)
                      n1110 = Compound Arithmetic op=OR(w1522, w1523, w1524, w1521, w1525, w1526, w1527, w1528, w1529, w1530, w1531, w1532, w1533, w1534, w1535) -> (w1520:bool)
                      "P2 position" <- w1520
                      n1111 = Index Array(array=w1566, index=0) -> (element=w1561:i32)
                      n1112 = Boolean To (0,1)(Boolean=w1554) -> (0, 1=w1518:i16)
                      n1113 = Select(t=w1561, s=w1554, f=w1563) -> (s? t:f=→"p1code":i32)
                      n1114 = Compound Arithmetic op=OR(w1520, w1557, w1515, w1514) -> (w1552:bool)
                      n1115 = Or(x=w1552, y=w1551) -> (x .or. y?=w1550:bool)
                      n1116 = local read "p2code"() -> (w1560:i32)
                      n1117 = Select(t=w1561, s=w1550, f=w1560) -> (s? t:f=→"p2code":i32)
                      n1118 = Boolean To (0,1)(Boolean=w1550) -> (0, 1=w1519:i16)
                    }
                    frame #3 {
                      n1119 = Build Array("1", "2", "3", "4", "5", "6", "7", "8", "9", "10", "1 2", "2 2", "3 2", "4 2", "5 2", "6 2", "7 2", "8 2", "9 2", "10 2") -> (w1621:bool[])
                      "FH" <- w1621
                      n1120 = Or Array Elements(Boolean array=w1621) -> (logical OR=w1611:bool)
                      n1121 = Boolean To (0,1)(Boolean=w1611) -> (0, 1=w1571:i16)
                      n1122 = Build Array("1 3", "2 3", "3 3", "4 3", "5 3", "6 3", "7 3", "8 3", "9 3", "10 3", "1 4", "2 4", "3 4", "4 4", "5 4", "6 4", "7 4", "8 4", "9 4", "10 4") -> (w1613:bool[])
                      "BH" <- w1613
                      n1123 = Or Array Elements(Boolean array=w1613) -> (logical OR=w1610:bool)
                      n1124 = Boolean To (0,1)(Boolean=w1610) -> (0, 1=w1570:i16)
                      n1125 = Build Array("1 5", "2 5", "3 5", "4 5", "5 5", "6 5", "7 5", "8 5", "9 5", "10 5", "1 6", "2 6", "3 6", "4 6", "5 6", "6 6", "7 6", "8 6", "9 6", "10 6") -> (w1612:bool[])
                      "OH" <- w1612
                      n1126 = Or Array Elements(Boolean array=w1612) -> (logical OR=w1609:bool)
                      n1127 = Boolean To (0,1)(Boolean=w1609) -> (0, 1=w1569:i16)
                    }
                    frame #4 {
                      w1694 = 10 ("index")
                      n1128 = local read "BH"() -> (w1686:bool[])
                      n1129 = local read "OH"() -> (w1685:bool[])
                      n1130 = local read "FH"() -> (w1687:bool[])
                      n1131 = Split 1D Array(array=w1687, index=w1694) -> (first subarray=w1683:bool[], second subarray=w1684:bool[])
                      n1132 = Split 1D Array(array=w1686, index=w1694) -> (first subarray=w1693:bool[], second subarray=w1691:bool[])
                      n1133 = Split 1D Array(array=w1685, index=w1694) -> (first subarray=w1692:bool[], second subarray=w1690:bool[])
                      n1134 = Build Array(w1683, w1693, w1692) -> (w1682:bool[][])
                      n1135 = Build Array(w1684, w1691, w1690) -> (w1681:bool[][])
                      n1136 = Or Array Elements(Boolean array=w1682) -> (logical OR=w1689:bool)
                      n1137 = Or Array Elements(Boolean array=w1681) -> (logical OR=w1688:bool)
                      n1138 = Insert Into Array(array=w1682, new element=w1681) -> (w1680:bool[][])  [unwired: 2 in]
                      n1139 = Boolean To (0,1)(Boolean=w1689) -> (0, 1=w1651:i16)
                      n1140 = Boolean To (0,1)(Boolean=w1688) -> (0, 1=w1650:i16)
                      n1141 = Index Array(array=w1680, index (col) #1=3 ("disabled index (col)"), index (col) #2=4 ("index (col)"), index (col) #3=2 ("index (col)"), index (col) #4=1 ("index (col)"), index (col) #5=6 ("index (col)"), index (col) #6=5 ("index (col)"), index (col) #7=0 ("index (col)"), index (col) #8=7 ("index (col)"), index (col) #9=8 ("index (col)"), index (col) #10=9 ("index (col)")) -> (element #1=w1670:bool[], element #2=w1662:bool[], element #3=w1661:bool[], element #4=w1660:bool[], element #5=w1659:bool[], element #6=w1658:bool[], element #7=w1657:bool[], element #8=w1656:bool[], element #9=w1639:bool[], element #10=w1638:bool[])  [unwired: 10 in]
                      n1142 = Or Array Elements(Boolean array=w1670) -> (logical OR=w1671:bool)
                      n1143 = Or Array Elements(Boolean array=w1661) -> (logical OR=w1667:bool)
                      n1144 = Or Array Elements(Boolean array=w1659) -> (logical OR=w1666:bool)
                      n1145 = Or Array Elements(Boolean array=w1657) -> (logical OR=w1663:bool)
                      n1146 = Or Array Elements(Boolean array=w1639) -> (logical OR=w1653:bool)
                      n1147 = Or Array Elements(Boolean array=w1662) -> (logical OR=w1669:bool)
                      n1148 = Or Array Elements(Boolean array=w1660) -> (logical OR=w1668:bool)
                      n1149 = Or Array Elements(Boolean array=w1658) -> (logical OR=w1665:bool)
                      n1150 = Or Array Elements(Boolean array=w1656) -> (logical OR=w1664:bool)
                      n1151 = Or Array Elements(Boolean array=w1638) -> (logical OR=w1652:bool)
                      n1152 = Boolean To (0,1)(Boolean=w1671) -> (0, 1=w1649:i16)
                      n1153 = Boolean To (0,1)(Boolean=w1667) -> (0, 1=w1647:i16)
                      n1154 = Boolean To (0,1)(Boolean=w1666) -> (0, 1=w1645:i16)
                      n1155 = Boolean To (0,1)(Boolean=w1663) -> (0, 1=w1643:i16)
                      n1156 = Boolean To (0,1)(Boolean=w1653) -> (0, 1=w1641:i16)
                      n1157 = Boolean To (0,1)(Boolean=w1669) -> (0, 1=w1648:i16)
                      n1158 = Boolean To (0,1)(Boolean=w1668) -> (0, 1=w1646:i16)
                      n1159 = Boolean To (0,1)(Boolean=w1665) -> (0, 1=w1644:i16)
                      n1160 = Boolean To (0,1)(Boolean=w1664) -> (0, 1=w1642:i16)
                      n1161 = Boolean To (0,1)(Boolean=w1652) -> (0, 1=w1640:i16)
                    }
                    frame #5 {
                      n1162 = local read "P2 position"() -> (w1709:bool)
                      n1163 = local read "P1 position"() -> (w1705:bool)
                      n1164 = local read "BH"() -> (w1703:bool[])
                      n1165 = local read "OH"() -> (w1704:bool[])
                      n1166 = local read "FH"() -> (w1702:bool[])
                      n1167 = Or(x="W2", y="E2") -> (x .or. y?=w1713:bool)
                      n1168 = Or(x="W1", y="E1") -> (x .or. y?=w1710:bool)
                      n1169 = Or Array Elements(Boolean array=w1703) -> (logical OR=w1707:bool)
                      n1170 = Or Array Elements(Boolean array=w1704) -> (logical OR=w1708:bool)
                      n1171 = Or Array Elements(Boolean array=w1702) -> (logical OR=w1706:bool)
                      n1172 = Compound Arithmetic op=OR(w1705, w1706, w1707, w1708, w1709) -> (invert w1712:bool)
                      n1173 = And(x=w1712, y=w1713) -> (x .and. y?=w1714:bool)
                      n1174 = And(x=w1712, y=w1710) -> (x .and. y?=w1711:bool)
                      n1175 = Boolean To (0,1)(Boolean=w1711) -> (0, 1=w1701:i16)
                      n1176 = Select(t=2.0, s=w1714, f=w1701) -> (s? t:f=w1696:dbl)
                      n1177 = case shown="2" w1696 {
                        tunnel: [w1715 w1744 w1747] -> _
                        frame 0, Default {
                          n1178 = local read "coding"() -> (w1715:i32[][])
                        }
                        frame 1 {
                          n1179 = local read "Score2"() -> (w1716:i32)
                          n1180 = local read "Score1"() -> (w1742:i32)
                          n1181 = local read "W1"() -> (w1738:bool)
                          n1182 = local read "W2"() -> (w1739:bool)
                          n1183 = local read "E1"() -> (w1740:bool)
                          n1184 = local read "E2"() -> (w1741:bool)
                          n1185 = Increment(x=w1716) -> (x+1=w1734:i32)
                          n1186 = Or(x=w1739, y=w1740) -> (x .or. y?=w1736:bool)
                          n1187 = Increment(x=w1742) -> (x+1=w1735:i32)
                          n1188 = Or(x=w1738, y=w1741) -> (x .or. y?=w1737:bool)
                          n1189 = Boolean To (0,1)(Boolean=w1738) -> (0, 1=w1730:i16)
                          n1190 = Boolean To (0,1)(Boolean=w1739) -> (0, 1=w1729:i16)
                          n1191 = Boolean To (0,1)(Boolean=w1740) -> (0, 1=w1724:i16)
                          n1192 = Boolean To (0,1)(Boolean=w1741) -> (0, 1=w1723:i16)
                          n1193 = Select(t=w1734, s=w1736, f=w1716) -> (s? t:f=w1717:i32)
                          n1194 = local read "p1code"() -> (w1732:i32)
                          n1195 = local read "coding"() -> (w1743:i32[][])
                          n1196 = Select(t=w1735, s=w1737, f=w1742) -> (s? t:f=w1719:i32)
                          n1197 = Boolean To (0,1)(Boolean=w1737) -> (0, 1=w1722:i16)
                          n1198 = Boolean To (0,1)(Boolean=w1736) -> (0, 1=w1721:i16)
                          n1199 = local write "Score1"(w1719) -> ()
                          n1200 = local write "Score2"(w1717) -> ()
                          n1201 = Replace Array Subset(array=w1743, new element #1=w1730, index (row) #1=w1732, index (col) #1=31 ("disabled index (col)"), new element #2=w1729, index (row) #2=w1732, index (col) #2=32 ("disabled index (col)"), new element #3=w1724, index (row) #3=w1732, index (col) #3=33 ("disabled index (col)"), new element #4=w1723, index (row) #4=w1732, index (col) #4=34 ("disabled index (col)"), new element #5=w1722, index (row) #5=w1732, index (col) #5=35 ("disabled index (col)"), new element #6=w1721, index (row) #6=w1732, index (col) #6=36 ("disabled index (col)"), new element #7=w1719, index (row) #7=w1732, index (col) #7=37 ("disabled index (col)"), new element #8=w1717, index (row) #8=w1732, index (col) #8=38 ("disabled index (col)")) -> (w1744:i32[][])
                          n1202 = local write "coding"(w1744) -> ()
                        }
                        frame 2 {
                          n1203 = local read "W1"() -> (w1769:bool)
                          n1204 = local read "W2"() -> (w1770:bool)
                          n1205 = local read "E1"() -> (w1771:bool)
                          n1206 = local read "E2"() -> (w1772:bool)
                          n1207 = Increment(x="Score1") -> (x+1=w1766:i32)
                          n1208 = Boolean To (0,1)(Boolean=w1769) -> (0, 1=w1762:i16)
                          n1209 = Boolean To (0,1)(Boolean=w1770) -> (0, 1=w1761:i16)
                          n1210 = Boolean To (0,1)(Boolean=w1771) -> (0, 1=w1756:i16)
                          n1211 = Boolean To (0,1)(Boolean=w1772) -> (0, 1=w1755:i16)
                          n1212 = Or(x=w1769, y=w1772) -> (x .or. y?=w1768:bool)
                          n1213 = Or(x=w1770, y=w1771) -> (x .or. y?=w1767:bool)
                          n1214 = Increment(x="Score2") -> (x+1=w1765:i32)
                          n1215 = Select(t=w1765, s=w1767, f="Score2") -> (s? t:f=w1749:i32)
                          n1216 = Select(t=w1766, s=w1768, f="Score1") -> (s? t:f=w1751:i32)
                          n1217 = Boolean To (0,1)(Boolean=w1768) -> (0, 1=w1754:i16)
                          n1218 = Boolean To (0,1)(Boolean=w1767) -> (0, 1=w1753:i16)
                          n1219 = local read "p2code"() -> (w1748:i32)
                          n1220 = local read "coding"() -> (w1773:i32[][])
                          n1221 = local write "Score1"(w1751) -> ()
                          n1222 = local write "Score2"(w1749) -> ()
                          n1223 = Replace Array Subset(array=w1773, new element #1=w1762, index (row) #1=w1748, index (col) #1=31 ("disabled index (col)"), new element #2=w1761, index (row) #2=w1748, index (col) #2=32 ("disabled index (col)"), new element #3=w1756, index (row) #3=w1748, index (col) #3=33 ("disabled index (col)"), new element #4=w1755, index (row) #4=w1748, index (col) #4=34 ("disabled index (col)"), new element #5=w1754, index (row) #5=w1748, index (col) #5=35 ("disabled index (col)"), new element #6=w1753, index (row) #6=w1748, index (col) #6=36 ("disabled index (col)"), new element #7=w1751, index (row) #7=w1748, index (col) #7=37 ("disabled index (col)"), new element #8=w1749, index (row) #8=w1748, index (col) #8=38 ("disabled index (col)")) -> (w1747:i32[][])
                          n1224 = local write "coding"(w1747) -> ()
                        }
                      }
                    }
                    frame #6 {
                      n1225 = Boolean To (0,1)(Boolean="1") -> (0, 1=w1786:i16)
                      n1226 = Boolean To (0,1)(Boolean="2") -> (0, 1=w1785:i16)
                      n1227 = Boolean To (0,1)(Boolean="3") -> (0, 1=w1784:i16)
                      n1228 = Boolean To (0,1)(Boolean="4") -> (0, 1=w1783:i16)
                      n1229 = Boolean To (0,1)(Boolean="5") -> (0, 1=w1782:i16)
                      n1230 = Boolean To (0,1)(Boolean="S1") -> (0, 1=w1792:i16)
                      n1231 = Boolean To (0,1)(Boolean="S2") -> (0, 1=w1791:i16)
                      n1232 = Boolean To (0,1)(Boolean="S3") -> (0, 1=w1788:i16)
                      n1233 = Boolean To (0,1)(Boolean="S4") -> (0, 1=w1787:i16)
                      n1234 = Boolean To (0,1)(Boolean="Player 1") -> (0, 1=w1777:i16)
                      n1235 = Boolean To (0,1)(Boolean="Player 2") -> (0, 1=w1776:i16)
                      n1236 = Boolean To (0,1)(Boolean="Player 3") -> (0, 1=w1775:i16)
                      n1237 = Boolean To (0,1)(Boolean="Player 4") -> (0, 1=w1774:i16)
                    }
                    frame #7 {
                      w1801 = FALSE ("4 6")
                      n1238 = local write "1 6"(w1801) -> ()
                      n1239 = local write "2 6"(w1801) -> ()
                      n1240 = local write "3 6"(w1801) -> ()
                      n1241 = local write "4 6"(w1801) -> ()
                      n1242 = local write "5 6"(w1801) -> ()
                      n1243 = local write "6 6"(w1801) -> ()
                      n1244 = local write "7 6"(w1801) -> ()
                      n1245 = local write "8 6"(w1801) -> ()
                      n1246 = local write "9 6"(w1801) -> ()
                      n1247 = local write "10 6"(w1801) -> ()
                      n1248 = local write "1 5"(w1801) -> ()
                      n1249 = local write "2 5"(w1801) -> ()
                      n1250 = local write "3 5"(w1801) -> ()
                      n1251 = local write "4 5"(w1801) -> ()
                      n1252 = local write "5 5"(w1801) -> ()
                      n1253 = local write "6 5"(w1801) -> ()
                      n1254 = local write "7 5"(w1801) -> ()
                      n1255 = local write "8 5"(w1801) -> ()
                      n1256 = local write "9 5"(w1801) -> ()
                      n1257 = local write "10 5"(w1801) -> ()
                      n1258 = local write "1 4"(w1801) -> ()
                      n1259 = local write "2 4"(w1801) -> ()
                      n1260 = local write "3 4"(w1801) -> ()
                      n1261 = local write "4 4"(w1801) -> ()
                      n1262 = local write "5 4"(w1801) -> ()
                      n1263 = local write "6 4"(w1801) -> ()
                      n1264 = local write "7 4"(w1801) -> ()
                      n1265 = local write "8 4"(w1801) -> ()
                      n1266 = local write "9 4"(w1801) -> ()
                      n1267 = local write "10 4"(w1801) -> ()
                      n1268 = local write "1 3"(w1801) -> ()
                      n1269 = local write "2 3"(w1801) -> ()
                      n1270 = local write "3 3"(w1801) -> ()
                      n1271 = local write "4 3"(w1801) -> ()
                      n1272 = local write "5 3"(w1801) -> ()
                      n1273 = local write "6 3"(w1801) -> ()
                      n1274 = local write "7 3"(w1801) -> ()
                      n1275 = local write "8 3"(w1801) -> ()
                      n1276 = local write "9 3"(w1801) -> ()
                      n1277 = local write "10 3"(w1801) -> ()
                      n1278 = local write "1 2"(w1801) -> ()
                      n1279 = local write "2 2"(w1801) -> ()
                      n1280 = local write "3 2"(w1801) -> ()
                      n1281 = local write "4 2"(w1801) -> ()
                      n1282 = local write "5 2"(w1801) -> ()
                      n1283 = local write "6 2"(w1801) -> ()
                      n1284 = local write "7 2"(w1801) -> ()
                      n1285 = local write "8 2"(w1801) -> ()
                      n1286 = local write "9 2"(w1801) -> ()
                      n1287 = local write "10 2"(w1801) -> ()
                      n1288 = local write "1"(w1801) -> ()
                      n1289 = local write "2"(w1801) -> ()
                      n1290 = local write "3"(w1801) -> ()
                      n1291 = local write "4"(w1801) -> ()
                      n1292 = local write "5"(w1801) -> ()
                      n1293 = local write "6"(w1801) -> ()
                      n1294 = local write "7"(w1801) -> ()
                      n1295 = local write "8"(w1801) -> ()
                      n1296 = local write "9"(w1801) -> ()
                      n1297 = local write "10"(w1801) -> ()
                      n1298 = local write "BCL 3"(w1801) -> ()
                      n1299 = local write "BCL 2"(w1801) -> ()
                      n1300 = local write "BL 3"(w1801) -> ()
                      n1301 = local write "BL 2"(w1801) -> ()
                      n1302 = local write "BC 3"(w1801) -> ()
                      n1303 = local write "BC 2"(w1801) -> ()
                      n1304 = local write "BCR 3"(w1801) -> ()
                      n1305 = local write "BCR 2"(w1801) -> ()
                      n1306 = local write "Player 1"(w1801) -> ()
                      n1307 = local write "Player 2"(w1801) -> ()
                      n1308 = local write "Player 3"(w1801) -> ()
                      n1309 = local write "Player 4"(w1801) -> ()
                      n1310 = local write "BR 2"(w1801) -> ()
                      n1311 = local write "BR 3"(w1801) -> ()
                      n1312 = local write "W1"(w1801) -> ()
                      n1313 = local write "W2"(w1801) -> ()
                      n1314 = local write "E1"(w1801) -> ()
                      n1315 = local write "E2"(w1801) -> ()
                      n1316 = local write "TCL 3"(w1801) -> ()
                      n1317 = local write "TCL 2"(w1801) -> ()
                      n1318 = local write "TL 3"(w1801) -> ()
                      n1319 = local write "TL 2"(w1801) -> ()
                      n1320 = local write "TC 2"(w1801) -> ()
                      n1321 = local write "TC 3"(w1801) -> ()
                      n1322 = local write "TCR 3"(w1801) -> ()
                      n1323 = local write "TCR 2"(w1801) -> ()
                      n1324 = local write "TR 2"(w1801) -> ()
                      n1325 = local write "TR 3"(w1801) -> ()
                      n1326 = local read "coding"() -> (w1802:i32[][])
                      n1327 = local write "MCL 3"(w1801) -> ()
                      n1328 = local write "MCL 2"(w1801) -> ()
                      n1329 = local write "ML 3"(w1801) -> ()
                      n1330 = local write "ML 2"(w1801) -> ()
                      n1331 = local write "MC 2"(w1801) -> ()
                      n1332 = local write "MC 3"(w1801) -> ()
                      n1333 = local write "MR  2"(w1801) -> ()
                      n1334 = local write "MR  3"(w1801) -> ()
                      n1335 = local write "MCR  3"(w1801) -> ()
                      n1336 = local write "MCR 2"(w1801) -> ()
                      n1337 = local write "S1"(w1801) -> ()
                      n1338 = local write "S2"(w1801) -> ()
                      n1339 = local write "S3"(w1801) -> ()
                      n1340 = local write "S4"(w1801) -> ()
                      n1341 = local write "1"(w1801) -> ()
                      n1342 = local write "2"(w1801) -> ()
                      n1343 = local write "3"(w1801) -> ()
                      n1344 = local write "4"(w1801) -> ()
                      n1345 = local write "5"(w1801) -> ()
                    }
                  }
                  n1346 = call "IMAQ Dispose"("Image"=w1398) -> ()  [unwired: 5 in, 1 out]
                  n1347 = Build Array(w1413, w1414, w1397, w1396, w1395, w1394, w1393, w1392, w1391, w1390, w1389, w1388, w1387, w1386, w1385, w1384, w1383, w1382, w1381, w1380, w1379, w1378, w1377, w1376, w1375, w1374, w1373, w1372, w1371, w1370, w1369, w1368, w1368, w1368, w1368, w1368, w1368, w1368, w1368, w1367, w1366, w1365, w1364, w1363, w1362, w1361, w1358, w1357, w1359, w1360, w1356, w1355, w1354, w1353) -> (w1406:i32[])
                  n1348 = Delete From Array(array=w1406, index=0) -> (array with subset deleted=w1404:i32[])  [unwired: 1 in, 1 out]
                  n1349 = Insert Into Array(array=w1400, new element=w1406) -> (w1401:i32[][])  [unwired: 2 in]
                  n1350 = Array Max & Min(array=w1404) -> (max value=w1403:i32)  [unwired: 3 out]
                  n1351 = Equal To 0?(x=w1403) -> (x = 0?=w1402:bool)
                  n1352 = Select(t=w1400, s=w1402, f=w1401) -> (s? t:f=w1399:i32[][])
                  n1353 = Index Array(array=w1399, index (col)=0 ("disabled index (col)")) -> (element=w1408:i32[])  [unwired: 1 in]
                  n1354 = Array Max & Min(array=w1408) -> (max value=→"Last coded":i32)  [unwired: 3 out]
                  n1355 = local write "coding"(w1399) -> ()
                }
              }
              n1356 = case shown="True" "Stop and save" {
                tunnel: [FALSE ("T button?") w1164] -> w1126
                frame False {
                }
                frame True {
                  n1357 = Two Button Dialog(message="You are about to stop the notation process", 2:"Stop and Save" ("Left Button Text (\"Yes\")")) -> (T button?=w1164:bool)  [unwired: 1 in]
                }
              }
              n1358 = Strip Path(path="Save data") -> (stripped path=w1133:path)  [unwired: 1 out]
              n1359 = call <vilib>:"Get File Extension.vi"("file"="Save data") -> ("filename without extension"=w1130:string)  [unwired: 7 in, 3 out]
              n1360 = Path To String(path=w1133) -> (string=w1134:string)
              n1361 = Concatenate Strings(w1134, "\\" ("string"), w1130, "(BStAT DATA).xls" ("string")) -> (w1135:string)
              n1362 = String To Path(string=w1135) -> (path=w1127:path)
              n1363 = call <vilib>:"Check if File or Folder Exists.vi"("path"=w1127) -> ("file or folder exists?"=w1129:bool)  [unwired: 8 in, 2 out]
            }
            n1364 = local read "F_frame"() -> (w1109:u32)
            n1365 = local read "S_frame"() -> (w1108:u32)
            n1366 = property on="Progress..." class="Slide (strict)"("Scale.Maximum"=w1109, "Scale.Minimum"=w1108, "Visible"=w1095) -> ()  [unwired: 2 in, 2 out]
            n1367 = Not(x=w1095) -> (.not. x?=w1096:bool)
            n1368 = property on="Drag control" class="Slide (strict)"("Visible"=w1096) -> ()  [unwired: 2 in, 2 out]
            n1369 = Path to Array of Strings(0:w1103) -> (2:w1104:string[])  [unwired: 1 out]
            n1370 = Array Size(array=w1104) -> (size(s)=w1105:i32)
            n1371 = Decrement(x=w1105) -> (x-1=w1106:i32)
            n1372 = Index Array(array=w1104, index=w1106) -> (element=w1102:string)
            n1373 = Build Array("Name 1", "Name 2", "Name 3", "Name 4") -> (w1088:string[])
            n1374 = call "EVENTS(SubVI).vi"() -> ("Events"=w1094:string)  [unwired: 1 in]
            n1375 = call "Doubles Events (SubVI).vi"("Singles Events"=w1094, "PLAYER NAMES"=w1088) -> ("Edited Events For Doubles"=w1093:string)
            n1376 = Concatenate Strings("avi file" ("string"), w1101, w1102, w1101, w1101, w1093) -> (w1084:string)
            n1377 = call "IMAQ AVI Close"("Avi Refnum"=w1099) -> ()  [unwired: 10 in, 1 out]
            n1378 = case shown="False" w1087 {
              tunnel: w1086 -> [w1122 w1124]
              tunnel: w1084 -> [w1119 _]
              tunnel: w1085 -> [w1117 w1123]
              frame False {
                n1379 = Open/Create/Replace File(file path (use dialog)=w1117, operation (0:open)=T3."create") -> (refnum out=w1120:refnum<file>)  [unwired: 4 in, 2 out]
                n1380 = Write to Text File(file (use dialog)=w1120, text=w1119) -> (refnum out=w1116:refnum<file>)  [unwired: 2 in, 2 out]
                n1381 = Close File(refnum=w1116) -> (path=w1115:path)  [unwired: 1 in, 1 out]
                n1382 = call-poly <vilib>:"Write To Spreadsheet File.vi"("append to file? (new file:F)"=TRUE, "2D data"=w1122, "file path (dialog if empty)"=w1115) -> ()  [unwired: 5 in, 1 out]
              }
              frame True {
                n1383 = call-poly <vilib>:"Write To Spreadsheet File.vi"("append to file? (new file:F)"=TRUE, "2D data"=w1124, "file path (dialog if empty)"=w1123) -> ()  [unwired: 5 in, 1 out]
              }
            }
            n1384 = property on="Last coded" class="DigNum (strict)"("Visible"=w1098) -> ()  [unwired: 2 in, 2 out]
            n1385 = property on="UNDO" class="Bool (strict)"("Visible"=w1098) -> ()  [unwired: 2 in, 2 out]
            n1386 = property on="playback speed" class="Slide (strict)"("Visible"=w1098) -> ()  [unwired: 2 in, 2 out]
            n1387 = property on="Progress..." class="Slide (strict)"("Visible"=w1098) -> ()  [unwired: 2 in, 2 out]
            n1388 = property on="playback speed" class="Slide (strict)"("Visible"=w1097) -> ()  [unwired: 2 in, 2 out]
            n1389 = property on="Last coded" class="DigNum (strict)"("Visible"=w1097) -> ()  [unwired: 2 in, 2 out]
            n1390 = property on="UNDO" class="Bool (strict)"("Visible"=w1097) -> ()  [unwired: 2 in, 2 out]
            "coding" <- i32[][] [] ("coding")
          }
        }
        "S_frame" <- w1044
        "F_frame" <- w1044
      }
    }
  }
